vi "Image-DO with Stage - Main_v1.vi"() -> ()   [LabVIEW 2021]
doc: "This program was written by Dr. Michael Everly in support of the research efforts of Dr. Garth Simpson. It provides integrated data acquisition while scanning of a Newport 3 axis rotation stage.. \n\nHardware Required:\nNewport Corp., ESP300 -- 3 axis translation controller with rotation stages.\nTektronix TDS 30xx Oscilloscope\n\n\nWritten by\n Dr. Michael Everly\n Instrumentation Scientist\n Department of Chemistry\n Purdue University\n West Lafayette, IN 47907\n\nCopyright© 2005, All Rights Reserved"
uses:
  Box/Zhang lab general/Software/Amy Imaging_New/Amy Imaging 12-09-2024/Amy Imaging 12-09-2024/Applications/Image-DO with Stage Scan/Support/Type Defs/Image-DO with Stage - Stage Position.ctl
  Box/Zhang lab general/Software/Amy Imaging_New/Amy Imaging 12-09-2024/Amy Imaging 12-09-2024/Applications/Image-DO with Stage Scan/Support/Type Defs/Image-DO with Stage - Imaging Parameters GUI.ctl
  Box/Zhang lab general/Software/Amy Imaging_New/Amy Imaging 12-09-2024/Amy Imaging 12-09-2024/Common/Amy Imager/Type Defs/Imager - Scan Pattern.ctl
  Box/Zhang lab general/Software/Amy Imaging_New/Amy Imaging 12-09-2024/Amy Imaging 12-09-2024/Common/Amy Imager/Type Defs/Imager - Axis Parameters.ctl
  Box/Zhang lab general/Software/Amy Imaging_New/Amy Imaging 12-09-2024/Amy Imaging 12-09-2024/Applications/Image-DO with Stage Scan/Support/Type Defs/Image-DO with Stage - Stage Parameters-Random GUI.ctl
  Box/Zhang lab general/Software/Amy Imaging_New/Amy Imaging 12-09-2024/Amy Imaging 12-09-2024/Applications/Image-DO with Stage Scan/Support/Type Defs/Image-DO with Stage - XY Stage Parameters.ctl
  Box/Zhang lab general/Software/Amy Imaging_New/Amy Imaging 12-09-2024/Amy Imaging 12-09-2024/Applications/Image-DO with Stage Scan/Support/Type Defs/Image-DO with Stage - Z Stage Parameters.ctl
  Box/Zhang lab general/Software/Amy Imaging_New/Amy Imaging 12-09-2024/Amy Imaging 12-09-2024/Applications/Image-DO with Stage Scan/Support/Program Ctrl/Image-DO with Stage - Exec Que.ctl
  Box/Zhang lab general/Software/Amy Imaging_New/Amy Imaging 12-09-2024/Amy Imaging 12-09-2024/Applications/Image-DO with Stage Scan/Support/Program Ctrl/Image-DO with Stage - Exec States.ctl
  Box/Zhang lab general/Software/Amy Imaging_New/Amy Imaging 12-09-2024/Amy Imaging 12-09-2024/Applications/Image-DO with Stage Scan/Support/Program Ctrl/Image-DO with Stage - Sys State.ctl
  <vilib>/Utility/miscctls.llb/LVRectTypeDef.ctl
  Box/Zhang lab general/Software/Amy Imaging_New/Amy Imaging 12-09-2024/Amy Imaging 12-09-2024/Applications/Image-DO with Stage Scan/Support/Type Defs/Image-DO with Stage - File Save Option.ctl
  Box/Zhang lab general/Software/Amy Imaging_New/Amy Imaging 12-09-2024/Amy Imaging 12-09-2024/Applications/Image-DO with Stage Scan/Support/Type Defs/Image-DO with Stage - XYZ Stage Parameters.ctl
  Box/Zhang lab general/Software/Amy Imaging_New/Amy Imaging 12-09-2024/Amy Imaging 12-09-2024/Common/Amy Imager/Type Defs/Imager - AO Scan Settings.ctl
  Box/Zhang lab general/Software/Amy Imaging_New/Amy Imaging 12-09-2024/Amy Imaging 12-09-2024/Common/Amy Imager/Type Defs/Imager - Scan Starting Point.ctl
  <vilib>/Utility/error.llb/DialogType.ctl
  <vilib>/numeric/Random Number (Range) DBL.vi
  <vilib>/Platform/browser.llb/Open URL in Default Browser (string).vi
panel:
  in  "Amy URL":string="Amy Instrument Facility "
  in  "Exit":bool
  in  "Main Tab":enum32{"I/O Config", "Image"}(tab)
  in  "DAQmx Static DO Lines":tag="Dev1/port1/line0:2"
  in  "Y-Mirror DAQmx AO Channel":tag="Dev1/ao1"
  in  "X-Mirror DAQmx AO Channel":tag="Dev1/ao0"
  in  "DAQmx DO Port":tag="Dev1/port0"
  in  "DAQmx AI Channels":T1(array[cluster])=[{"DAQmx AI Channel"="Dev1/ai0", "Channel/Image Name"="Sample"}, {"DAQmx AI Channel"="Dev1/ai1", "Channel/Image Name"="Reference"}]
  in  "Max Value":dbl=1.0 format="%0.2f"
  in  "Min Value":dbl format="%0.2f"
  in  "Prior Stage VISA Resource":refnum<visa-resource-name>="COM1"
  in  "Connect":bool
  in  "Save Masks":bool
  in  "Common Mask":bool caption="Use Common Mask"
  in  "Get Masks":bool
  in  "Scan":bool
  in  "Get Image Mask":bool
  in  "Aquire Image":bool
  in  "Save Image":bool
  in  "Auto Save":bool
  in  "Path":path
  in  "Base Filename":string
  in  "Advance":bool
  in  "Images":dbl[][][](array[numeric])
  in  "Operation":enum32{"Imaging", "Stage Scan"}(tab)
  in  "Imageing Parameters":T2={"Sample Rate"=1000000.0, "Pattern"=enum."Unidirectional Raster", "X Mirror"={"# Pixels"=512, "Center"=0.0, "Span"=0.1, "# Points / Pixel"=10, "Pre-Line pts"=10, "Post-Line pts"=10}, "Y Mirror"={"# Pixels"=512, "Center"=0.0, "Span"=0.1, "# Points / Pixel"=1, "Pre-Line pts"=10, "Post-Line pts"=0}, "Averaged"=TRUE, "Active DO lines"={"Pixel Pattern Bit (0)"=FALSE, "Change Pixel Bit (1)"=FALSE, "New Line Bit (2)"=FALSE, "In Image Bit (3)"=FALSE, "Image Pattern Bits (4-7)"=FALSE}, "Statice DO"=[FALSE, FALSE, FALSE, FALSE, FALSE, FALSE, FALSE, FALSE]} caption="Imaging Parameters" {"Y Mirror"."Post-Line pts" min=0; "Y Mirror"."Pre-Line pts" min=0; "Y Mirror"."# Points / Pixel" min=1; "Y Mirror"."Span" min=0.0 max=0.0 format="%.3f"; "Y Mirror"."Center" format="%.3f"; "Y Mirror"."# Pixels" min=2; "X Mirror"."Post-Line pts" min=0; "X Mirror"."Pre-Line pts" min=0; "X Mirror"."# Points / Pixel" min=1; "X Mirror"."Span" min=0.0 max=0.0 format="%.3f"; "X Mirror"."Center" format="%.3f"; "X Mirror"."# Pixels" min=2}
  out "Estmated Frame Time":dbl caption="Estmated Time: Image / Frame" min=0.0 max=0.0 format="%.1f"
  in  "Cycle Time (sec)":dbl caption="Center" format="%.1f"
  in  "Dwell Time (sec)":dbl caption="Center" format="%.1f"
  in  "User Defined Points":T5={"Step Position"={"X Pos"=0.0, "Y Pos"=0.0, "Z Pos"=0.0}, "Status"="Empty", "First"=FALSE, "Back"=FALSE, "Next"=FALSE, "Last"=FALSE, "Insert Current"=FALSE, "Go To"=FALSE, "Delete"=FALSE, "Clear"=FALSE, "New Position"={"X Pos"=0.0, "Y Pos"=0.0, "Z Pos"=0.0}, "Insert"=FALSE} {"Step Position"."X Pos" format="%.1f"; "Step Position"."Y Pos" format="%.1f"; "Step Position"."Z Pos" format="%.1f"; "New Position"."X Pos" format="%.1f"; "New Position"."Y Pos" format="%.1f"; "New Position"."Z Pos" format="%.1f"}
  in  "Grid Parameters":T7={"X Axis"={"Start Pt"=0.0, "Step Size"=100.0, "# Steps"=12}, "Y Axis"={"Start Pt"=20.0, "Step Size"=2.0, "# Steps"=2}, "Pattern"=enum."Bidirectional Raster", "Major Axis"=FALSE} caption="X Axis" {"X Axis"."Step Size" format="%.1f"; "X Axis"."Start Pt" format="%.1f"; "X Axis"."# Steps" min=1 step=1; "Y Axis"."Step Size" format="%.1f"; "Y Axis"."Start Pt" format="%.1f"; "Y Axis"."# Steps" min=1 step=1}
  in  "XY Scan Mode":bool caption="Z Axis"
  in  "Z Scan Parameters":T8={"Z Axis"={"Start Pt"=100.0, "Step Size"=20.0, "# Steps"=0}, "Pattern"=enum."Unidirectional Raster", "Active"=FALSE} caption="X Axis" {"Z Axis"."Step Size" format="%.1f"; "Z Axis"."Start Pt" format="%.1f"; "Z Axis"."# Steps" min=1 step=1}
  in  "Step Mode":bool
  in  "Row #":dbl(c297)
  out "Status":string
  out "Current Position":T6 caption="Stage Position" {"X Pos" format="%.1f"; "Y Pos" format="%.1f"; "Z Pos" format="%.1f"}
  in  "Reset I/O":bool
  in  "Get Position":bool
  in  "Go Home Prior":bool
  in  "Set Home Prior":bool
  # "Static Digital Control Lines"
  # "Mirror Control"
  # "Digital / Mask Control"
  # "Image / Data Acquisition"
  # "Stage Control"
  # "Stage Scanning"
  # "Image Scanning"
  # "1         line #         8"
  # "Scanning Parameters"
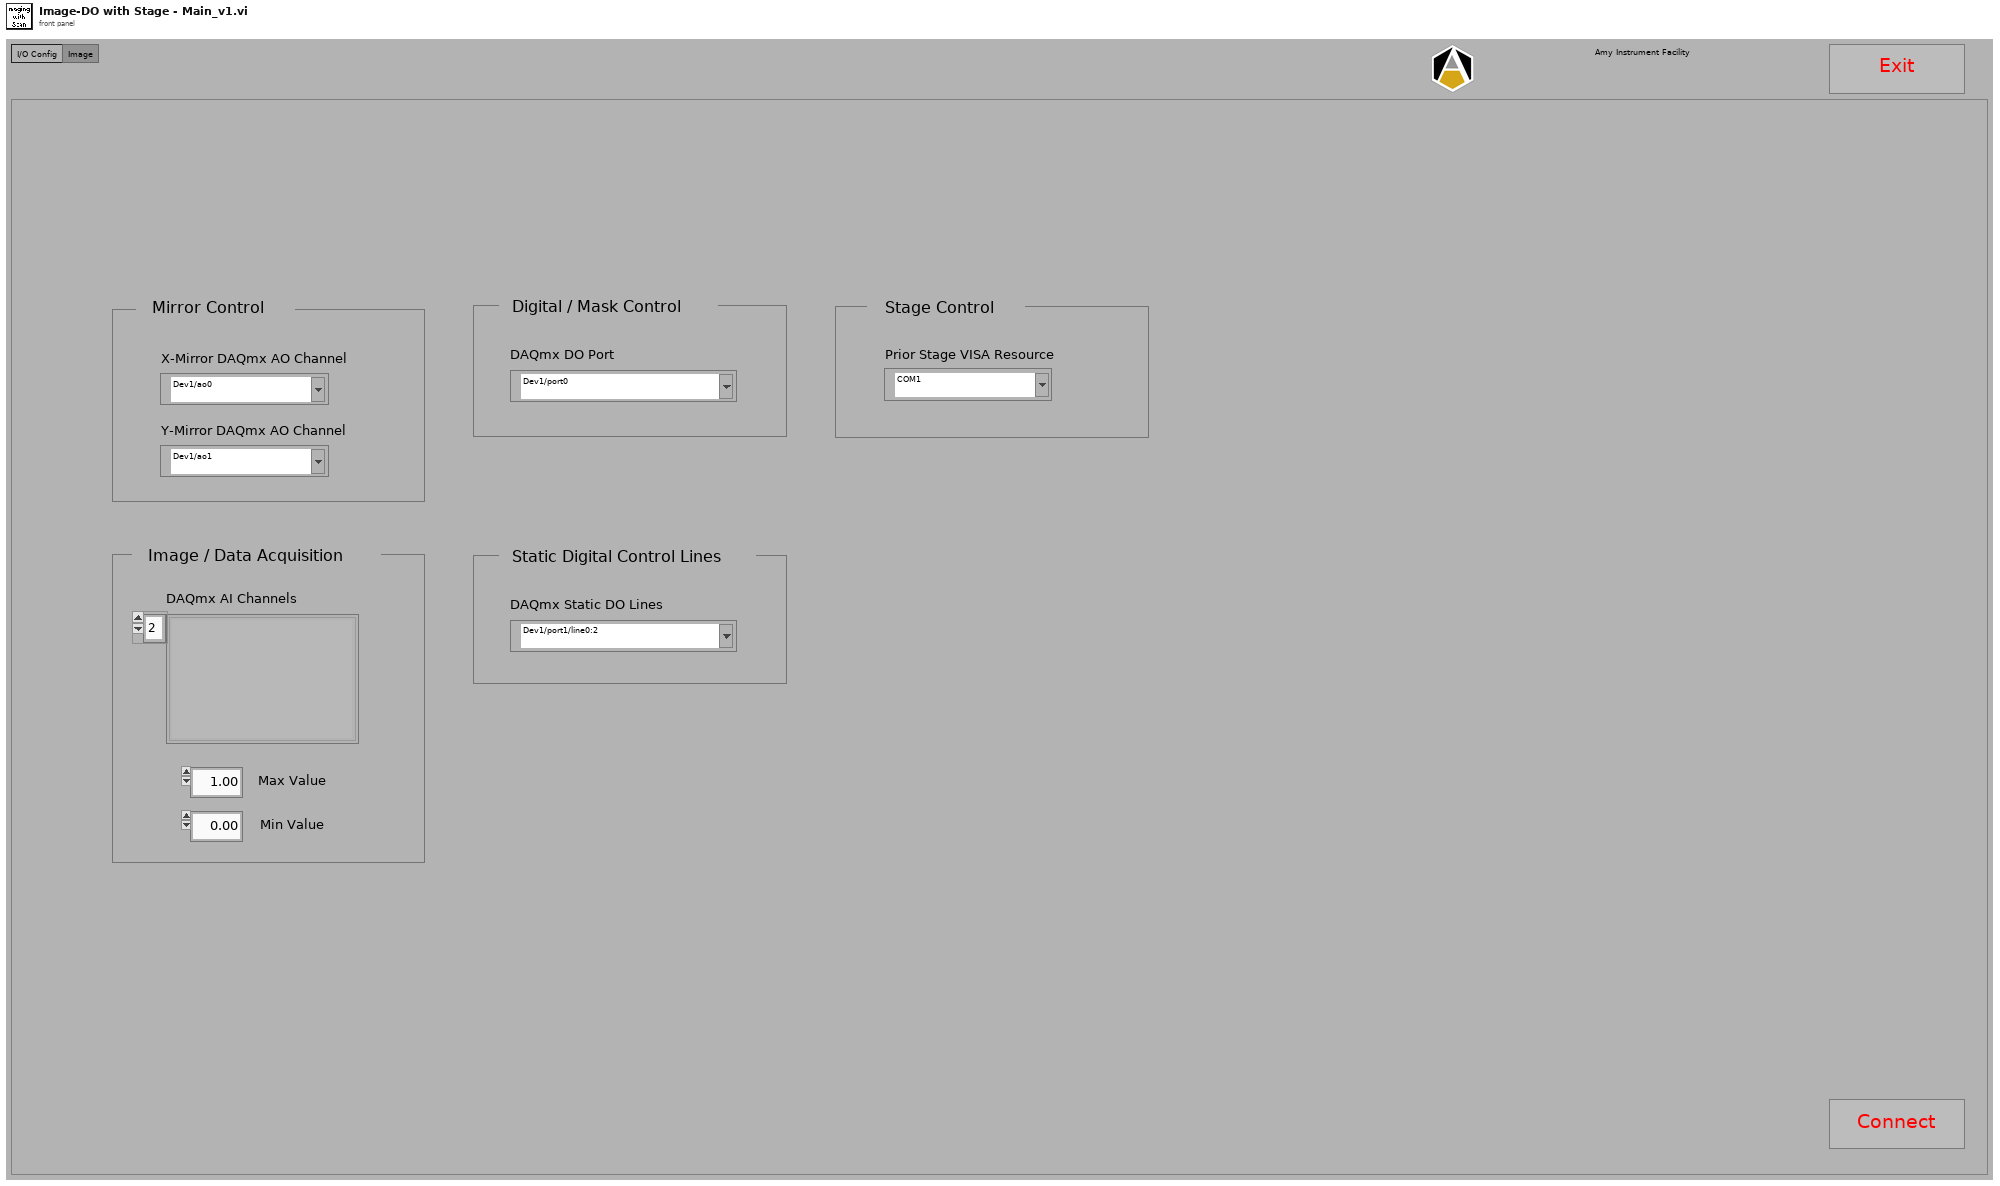
[diagram p1: front panel]
types:
  T1 = cluster{"DAQmx AI Channel":tag, "Channel/Image Name":string}[]
  T2 = typedef "Image-DO with Stage - Imaging Parameters GUI.ctl" = cluster{"Sample Rate":dbl, "Pattern":T3, "X Mirror":T4, "Y Mirror":T4, "Averaged":bool, "Active DO lines":cluster{"Pixel Pattern Bit (0)":bool, "Change Pixel Bit (1)":bool, "New Line Bit (2)":bool, "In Image Bit (3)":bool, "Image Pattern Bits (4-7)":bool}, "Statice DO":bool[]}
  T3 = typedef "Imager - Scan Pattern.ctl" = enum16{"Unidirectional Raster", "Bidirectional Raster"}
  T4 = typedef "Imager - Axis Parameters.ctl" = cluster{"# Pixels":i32, "Center":dbl, "Span":dbl, "# Points / Pixel":i32, "Pre-Line pts":i32, "Post-Line pts":i32}
  T5 = typedef "Image-DO with Stage - Stage Parameters-Random GUI.ctl" = cluster{"Step Position":T6, "Status":string, "First":bool, "Back":bool, "Next":bool, "Last":bool, "Insert Current":bool, "Go To":bool, "Delete":bool, "Clear":bool, "New Position":T6, "Insert":bool}
  T6 = typedef "Image-DO with Stage - Stage Position.ctl" = cluster{"X Pos":dbl, "Y Pos":dbl, "Z Pos":dbl}
  T7 = typedef "Image-DO with Stage - XY Stage Parameters.ctl" = cluster{"X Axis":cluster{"Start Pt":dbl, "Step Size":dbl, "# Steps":i32}, "Y Axis":cluster{"Start Pt":dbl, "Step Size":dbl, "# Steps":i32}, "Pattern":enum16{"Unidirectional Raster", "Bidirectional Raster"}, "Major Axis":bool}
  T8 = typedef "Image-DO with Stage - Z Stage Parameters.ctl" = cluster{"Z Axis":cluster{"Start Pt":dbl, "Step Size":dbl, "# Steps":i32}, "Pattern":enum16{"Unidirectional Raster", "Bidirectional Raster"}, "Active":bool}
  T9 = typedef "Image-DO with Stage - Exec Que.ctl" = cluster{"Exec States":T10, "U32":u32, "I32":i32, "DBL_1 (X)":dbl, "DBL_2 (Y)":dbl, "DBL_3 (Z)":dbl, "Bool_1":bool, "Bool_2":bool, "Variant":variant}
  T10 = typedef "Image-DO with Stage - Exec States.ctl" = enum16{"SW Init", "HW Init Ctrl", "HW Init - DAQmx", "HW Init - Prior", "HW Init - Reserve 1", "HW Init - Reserve 2", "HW Init - SW", "Pre-Image Crtl", "Pre-Image HW - DAQmx", "Pre-Image HW - Prior", "Pre-Image HW - Reserve 1", "Pre-Image HW - Reserve 2", "Pre-Image SW", "Image Ctrl", "Post-Image Crtl", "Post-Image HW - DAQmx", "Post-Image HW - Prior", "Post-Image HW - Reserve 1", "Post-Image HW - Reserve 2", "Post-Image SW", "Pre-Mask Ctrl", "Pre-Mask HW - DAQmx", "Pre-Mask HW - Prior", "Pre-Mask HW - Reserved 1", "Pre-Mask HW - Reserved 2", "Pre-Mask SW", "Mask Crtl", "Post-Mask Crtl", "Post-Mask HW - DAQmx", "Post-Mask HW - Prior", "Post-Mask HW - Reserved 1", "Post-Mask HW - Reserved 2", "Post-Mask SW", "Pre-Scan Ctrl", "Pre-Scan HW - DAQmx", "Pre-Scan HW - Prior", "Pre-Scan HW - Reserve 1", "Pre-Scan HW - Reserve 2", "Pre-Scan SW", "Scan Ctrl", "Post-Scan Crtl", "Post-Scan HW - DAQmx", "Post-Scan HW - Prior", "Post-Scan HW - Reserve 1", "Post-Scan HW - Reserve 2", "Post-Scan SW", "Wait (ms)", "Confgure Imaging - DAQmx", "Start Imaging - DAQmx", "Read Images - DAQmx", "Wait on Image Complete - DAQmx", "Stop Imaging - DAQmx", "Set Position - Prior", "Get Position - Prior", "Wait on Move Complete - Prior", "Process Data", "Display Image", "Display Scan", "Save Files", "Wait on User", "Update Mask", "Reserved 3", "Reserved 4", "Reserved 5", "HW Close Crtl", "HW Close - DAQmx", "HW Close - Prior", "HW Close - Reserve 1", "HW Close - Reserve 2", "HW Close - SW", "Shutdown", "Error", "Exit"}
  T11 = enum16{"Get All", "Set Path", "Set Filename", "Set Descriptor", "Set Image Settings", "Set Stage Settings", "Set # XY Points"}
  T12 = typedef "Image-DO with Stage - Sys State.ctl" = enum16{"HW Un_init", "HW Initializing", "HW Initialized", "Configuring", "Configured", "Imaging", "Masking", "Scanning"}
  T13 = cluster{"Exec States":u16, "U32":u32, "I32":i32, "DBL_1 (X)":dbl, "DBL_2 (Y)":dbl, "DBL_3 (Z)":dbl, "Bool_1":bool, "Bool_2":bool, "Variant":variant}[]
  T14 = enum16{"Read", "Go to First", "Step Forward", "Step Back", "Go to Last", "Insert", "Delete", "Delete All", "Insert Pts in"}
  T15 = typedef "Image-DO with Stage - File Save Option.ctl" = enum16{"Save Image Parameters", "Save Scan Parameters", "Save Mask", "Save Image", "Open Data Files", "Append Data Files", "Close Data Files"}
  T16 = typedef "Image-DO with Stage - Imaging Settings.ctl" = cluster{"DAQmx AI Channels":tag[], "Channel Names":string[], "Sample Rate":dbl, "Pattern":T3, "Starting Pt":T17, "X Mirror":T4, "Y Mirror":T4, "Averaged Data":bool}
  T17 = typedef "Imager - Scan Starting Point.ctl" = enum16{"X-Min, Y-Min", "X-Min, Y-Max", "X-Max, Y-Min", "X-Max, Y-Max"}
  T18 = cluster{"Step Position":cluster{"X Pos":bool, "Y Pos":bool, "Z Pos":bool}, "Status":bool, "First":bool, "Back":bool, "Next":bool, "Last":bool, "Insert Current":bool, "Go To":bool, "Delete":bool, "Clear":bool, "New Position":cluster{"X Pos":bool, "Y Pos":bool, "Z Pos":bool}, "Insert":bool}
  T19 = enum16{"Get All Mask", "Set Imaging Mask", "Init Scan Masks", "Get Scan Mask (n)", "Set Scan Mask (n)", "Set Scan Masks"}
  T20 = typedef "LVRectTypeDef.ctl" = cluster{"Left":i16, "Top":i16, "Right":i16, "Bottom":i16}
  T21 = enum16{"Create Task", "Write Lnes", "Clear Task"}
  T22 = enum16{"Get Current", "Go Home/First", "Step Forward", "Step Back", "Go To #", "Load Points"}
  T23 = typedef "Image-DO with Stage - XYZ Stage Parameters.ctl" = cluster{"Grid":T7, "Z Scan":T8, "XY Scan Mode":bool, "Dwell Time":dbl, "Cycle Time":dbl}
  T24 = typedef "Imager - AO Scan Settings.ctl" = cluster{"Sample Rate":dbl, "Pattern":T3, "Starting Pt":T17, "X Mirror":T4, "Y Mirror":T4}
  T25 = cluster{"DO Port Map":cluster{"Pixel Pattern Bit (0)":u8, "Change Pixel Bit (1)":u8, "New Line Bit (2)":u8, "In Image Bit (3)":u8, "Image Pattern Bits (4-7)":u8}, "Active DO lines":cluster{"Pixel Pattern Bit (0)":bool, "Change Pixel Bit (1)":bool, "New Line Bit (2)":bool, "In Image Bit (3)":bool, "Image Pattern Bits (4-7)":bool}, "Pixel Mask":u8[][], "Image Mask":u8[][]}
  T26 = cluster{"X Axis":dbl, "Y Axis":dbl, "Z Axis":dbl}
  T27 = enum16{"Do not append", "Current File", "Alternate File"}
  T28 = typedef "Image-DO with Stage - Scan Step Info.ctl" = cluster{"# X Steps":i32, "# Y Steps":i32, "# Z Steps":i32, "# XY Steps":i32, "# Total Steps":i32, "X Step #":i32, "Y Step #":i32, "Z Step #":i32, "XY Step #":i32, "Total Step #":i32}
  T29 = cluster{"# XY Steps":i32, "# Pixels":i32, "# Pixels":i32}
  T30 = cluster{"Pixel Pattern Bit (0)":bool, "Change Pixel Bit (1)":bool, "New Line Bit (2)":bool, "In Image Bit (3)":bool, "Image Pattern Bits (4-7)":bool}
  T31 = typedef "DialogType.ctl" = u16
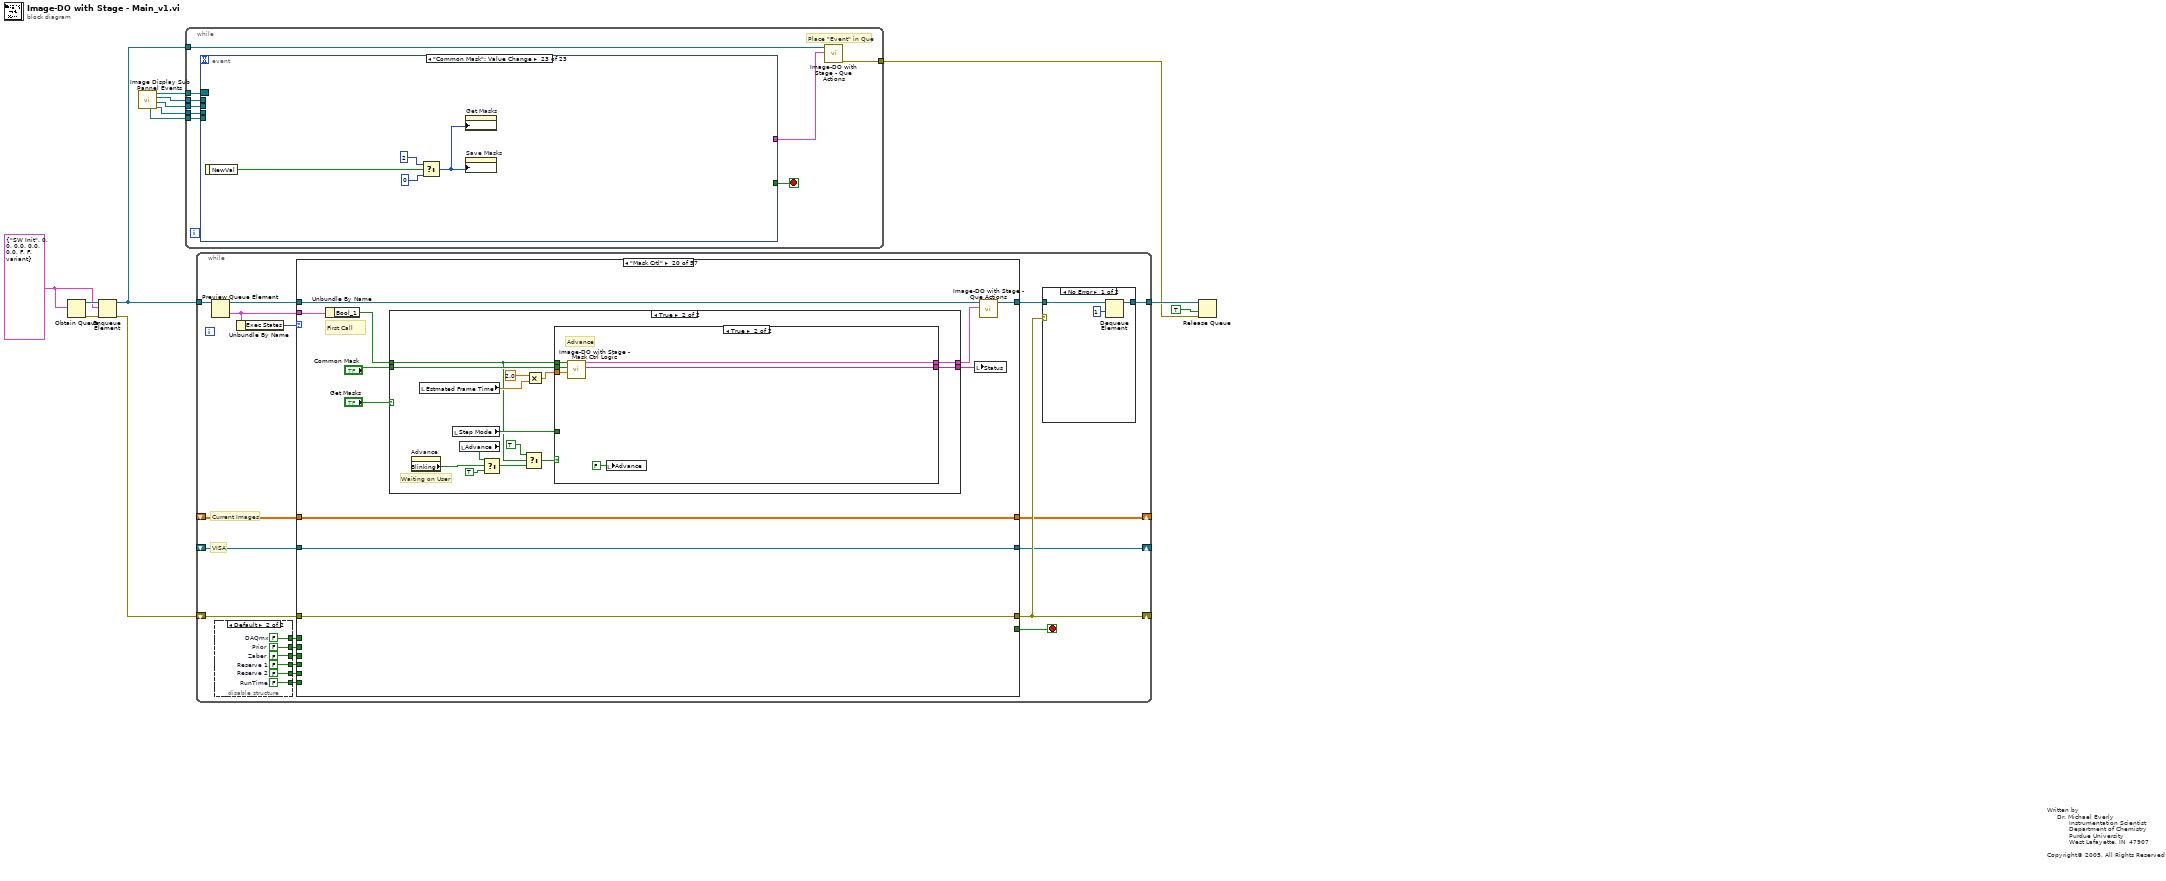
[diagram p0: block diagram]
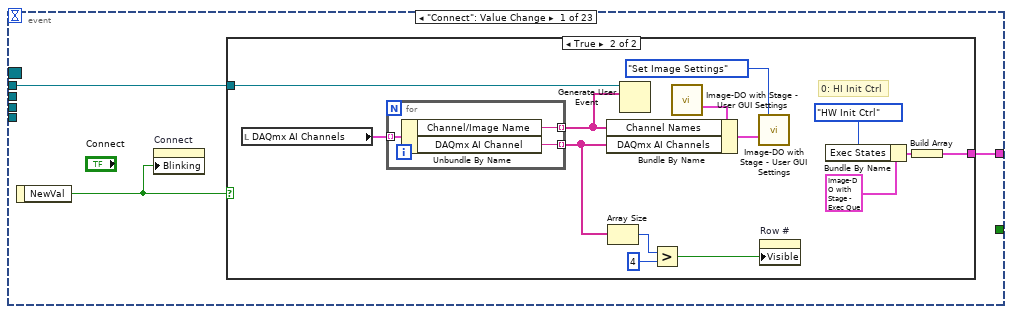
[diagram p2: hidden frame]
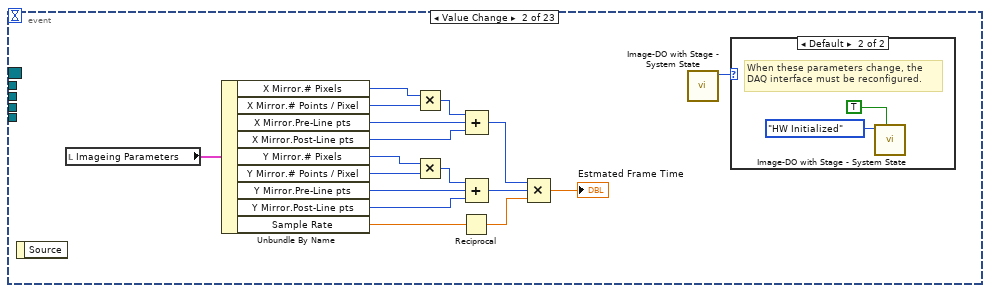
[diagram p4: hidden frame]
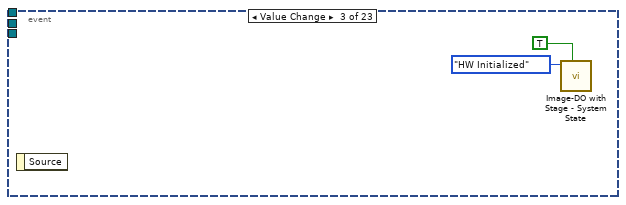
[diagram p6: hidden frame]
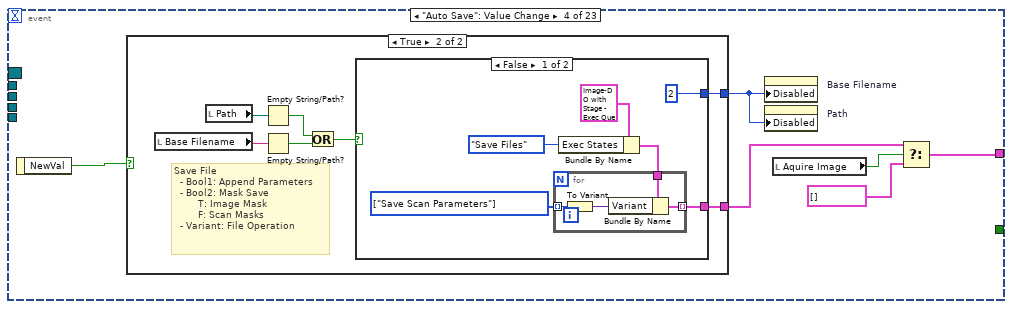
[diagram p7: hidden frame]
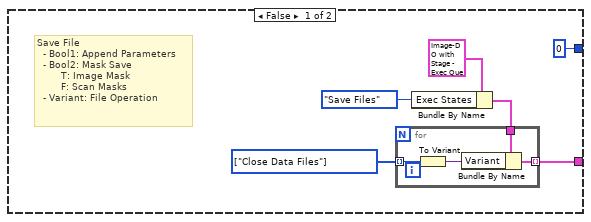
[diagram p8: hidden frame]
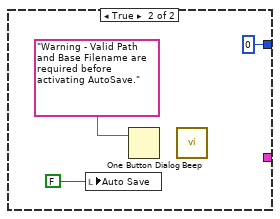
[diagram p9: hidden frame]
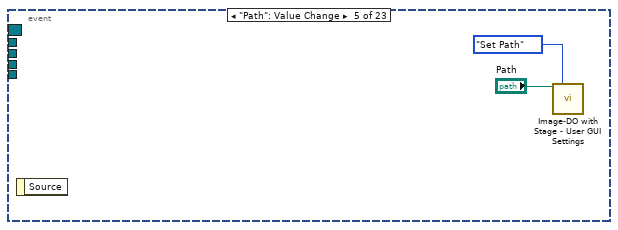
[diagram p10: hidden frame]
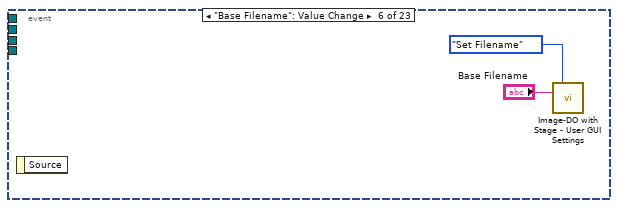
[diagram p11: hidden frame]
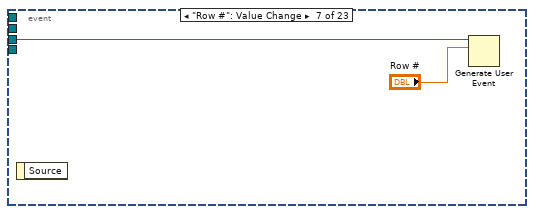
[diagram p12: hidden frame]
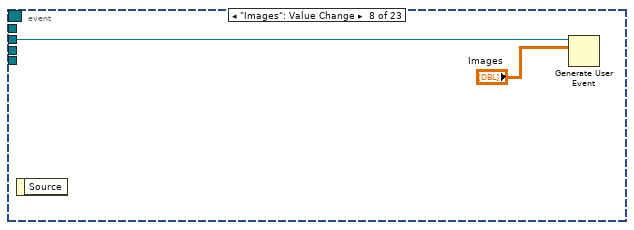
[diagram p13: hidden frame]
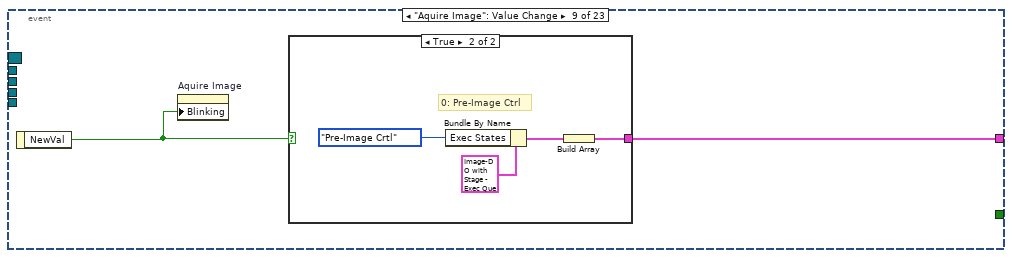
[diagram p14: hidden frame]
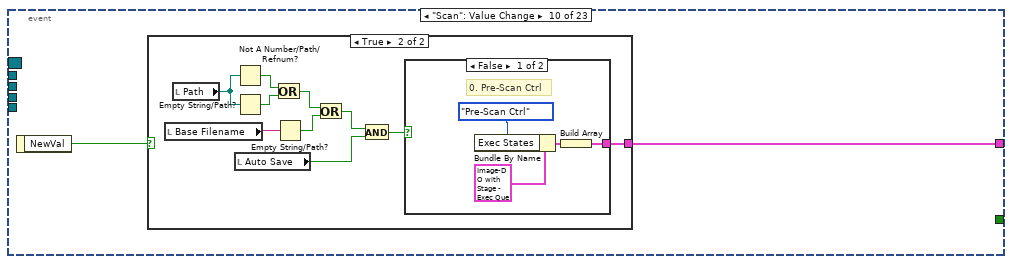
[diagram p16: hidden frame]
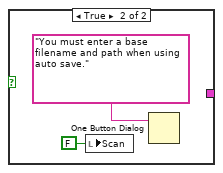
[diagram p18: hidden frame]
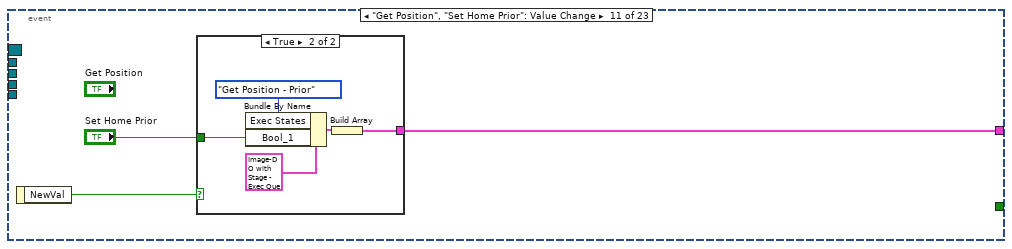
[diagram p19: hidden frame]
diagram:
  w9 = T9 {"Exec States"=enum."SW Init", "U32"=0, "I32"=0, "DBL_1 (X)"=0.0, "DBL_2 (Y)"=0.0, "DBL_3 (Z)"=0.0, "Bool_1"=FALSE, "Bool_2"=FALSE, "Variant"=variant(string "")}
  # "Written by\n     Dr. Michael Everly\n           Instrumentation Scientist\n           Department of Chemistry\n           Purdue University\n           West Lafayette, IN  47907\n\nCopyright© 2005, All Rights Reserved"
  n1 = Obtain Queue(element data type=w9) -> (queue out=w12:refnum<queue>, error out=w13:errorcluster)  [unwired: 4 in, 1 out]
  n2 = Enqueue Element(queue=w12, element=w9, error in (no error)=w13) -> (queue out=w10:refnum<queue>, error out=w11:errorcluster)  [unwired: 1 in, 1 out]
  n3 = call "Image Display Sub Pannel Events.vi"() -> ("Row # user event"=w2:refnum<user-event>, "Data user event"=w3:refnum<user-event>, "Captions user event"=w4:refnum<user-event>, "Event Registration Refnum"=w5:refnum<event-registration>, "Exit event out"=w1:refnum<user-event>)  [unwired: 7 in]
  n4 = while {
    tunnel: w10 -> [w21]
    tunnel: [w20] -> w6
    tunnel: w5 -> [w18]
    tunnel: w4 -> [w17]
    tunnel: w3 -> [w16]
    tunnel: w2 -> [w15]
    tunnel: w1 -> [w14]
    stop <- w19 stop-if-true
    # "Place \"Event\" in Que"
    n5 = event shown="[22] \"Common Mask\": Value Change" {
      selector: w18 -> [_ _ _ _ _ _ _ _ _ _ _ _ _ _ _ _ _ _ _ _ _ _ _]
      dyn-events: _ -> [_ _ _ _ _ _ _ _ _ _ _ _ _ _ _ _ _ _ _ _ _ _ _]
      timeout: _ -> [_ _ _ _ _ _ _ _ _ _ _ _ _ _ _ _ _ _ _ _ _ _ _]
      tunnel: [w25 _ _ w65 _ _ _ _ w108 w115 w134 w141 w151 w158 w167 _ _ _ w188 w248 w254 w261 _] -> w22
      tunnel: [_ _ _ _ _ _ _ _ _ _ _ _ _ _ w166 _ _ _ _ _ _ _ _] -> w19
      tunnel: w17 -> [w23 _ _ _ _ _ _ _ _ _ _ _ _ _ _ _ _ _ _ _ _ _ _]
      tunnel: w16 -> [_ _ _ _ _ _ _ w107 _ _ _ _ _ _ _ _ _ _ _ _ _ _ _]
      tunnel: w15 -> [_ _ _ _ _ _ w105 _ _ _ _ _ _ _ _ _ _ _ _ _ _ _ _]
      tunnel: w14 -> [_ _ _ _ _ _ _ _ _ _ _ _ _ _ w168 _ _ _ _ _ _ _ _]
      event "Connect": Value Change {
        n6 = event-data() -> ("NewVal"=w24:bool)  [unwired: 1 in]
        n7 = property on="Connect" class="Bool (strict)"("Blinking"=w24) -> ()  [unwired: 2 in, 2 out]
        n8 = case shown="True" w24 {
          tunnel: [_ w36] -> w25
          tunnel: w23 -> [_ w35]
          frame False {
          }
          frame True {
            # "0: HI Init Ctrl"
            n9 = local read "DAQmx AI Channels"() -> (w34:T1)
            n10 = for {
              tunnel: w34 -> [w42] mode=indexing
              tunnel: [w41] -> w33 mode=indexing
              tunnel: [w40] -> w30 mode=indexing
              n11 = Unbundle By Name(w42) -> ("Channel/Image Name"=w41:string, "DAQmx AI Channel"=w40:tag)
            }
            n12 = Array Size(array=w30) -> (size(s)=w32:i32)
            n13 = Generate User Event(user event=w35, event data cluster=w33) -> ()  [unwired: 2 in, 2 out]
            n14 = Greater?(x=w32, y=4) -> (0:w29:bool)
            n15 = call "Image-DO with Stage - User GUI Settings.vi"() -> ("Imaging Settings Out"=w27:T16)  [unwired: 10 in, 5 out]
            n16 = Bundle By Name(cluster=w27, "Channel Names"=w33, "DAQmx AI Channels"=w30) -> (w26:T16)
            n17 = call "Image-DO with Stage - User GUI Settings.vi"("Action (0: Read All)"=T11."Set Image Settings", "Imaging Settings In"=w26) -> ()  [unwired: 8 in, 6 out]
            n18 = property on="Row #" class="Scroll (strict)"("Visible"=w29) -> ()  [unwired: 2 in, 2 out]
            n19 = Bundle By Name(cluster=T9 {"Exec States"=enum."SW Init", "U32"=0, "I32"=0, "DBL_1 (X)"=0.0, "DBL_2 (Y)"=0.0, "DBL_3 (Z)"=0.0, "Bool_1"=FALSE, "Bool_2"=FALSE, "Variant"=variant(string "")} ("Que"), "Exec States"=Image-DO_with_Stage_-_Exec_States."HW Init Ctrl") -> (w39:T9)
            n20 = Build Array(w39) -> (w36:T9[])
          }
        }
      }
      event Value Change {
        n21 = event-data() -> ()  [unwired: 1 in, 1 out]
        n22 = local read "Imageing Parameters"() -> (w49:T2)
        n23 = Unbundle By Name(w49) -> ("X Mirror.# Pixels"=w51:i32, "X Mirror.# Points / Pixel"=w59:i32, "X Mirror.Pre-Line pts"=w57:i32, "X Mirror.Post-Line pts"=w56:i32, "Y Mirror.# Pixels"=w48:i32, "Y Mirror.# Points / Pixel"=w47:i32, "Y Mirror.Pre-Line pts"=w46:i32, "Y Mirror.Post-Line pts"=w45:i32, "Sample Rate"=w44:dbl)
        n24 = Multiply(x=w51, y=w59) -> (x*y=w58:i32)
        n25 = Multiply(x=w48, y=w47) -> (x*y=w55:i32)
        n26 = Reciprocal(x=w44) -> (1/x=w52:dbl)
        n27 = Compound Arithmetic op=ADD(w58, w57, w56) -> (w54:i32)
        n28 = Compound Arithmetic op=ADD(w55, w46, w45) -> (w53:i32)
        n29 = Compound Arithmetic op=MULTIPLY(w54, w53, w52) -> (→"Estmated Frame Time":dbl)
        n30 = call "Image-DO with Stage - System State.vi"() -> ("Sys State Out"=w43:T12)  [unwired: 9 in, 2 out]
        n31 = case shown="Default" w43 {
          frame "HW Un_init" {
          }
          frame Default {
            # "When these parameters change, the \nDAQ interface must be reconfigured."
            n32 = call "Image-DO with Stage - System State.vi"("Set State (F:Get)"=TRUE ("Action (F:Get)"), "Sys State In"=Image-DO_with_Stage_-_Sys_State."HW Initialized") -> ()  [unwired: 7 in, 3 out]
          }
        }
      }
      event Value Change {
        n33 = event-data() -> ()  [unwired: 1 in, 1 out]
        n34 = call "Image-DO with Stage - System State.vi"("Set State (F:Get)"=TRUE ("Action (F:Get)"), "Sys State In"=Image-DO_with_Stage_-_Sys_State."HW Initialized") -> ()  [unwired: 7 in, 3 out]
      }
      event "Auto Save": Value Change {
        n35 = event-data() -> ("NewVal"=w69:bool)  [unwired: 1 in]
        n36 = case shown="True" w69 {
          tunnel: [w71 w83] -> w67
          tunnel: [u8 0 ("Disabled") w80] -> w64
          frame False {
            w74 = T15[] [enum."Close Data Files"] items=["Save Image Parameters", "Save Scan Parameters", "Save Mask", "Save Image", "Open Data Files", "Append Data Files", "Close Data Files"]
            # "Save File\n  - Bool1: Append Parameters\n  - Bool2: Mask Save\n        T: Image Mask\n        F: Scan Masks\n  - Variant: File Operation"
            n37 = Bundle By Name(cluster=T9 {"Exec States"=enum."SW Init", "U32"=0, "I32"=0, "DBL_1 (X)"=0.0, "DBL_2 (Y)"=0.0, "DBL_3 (Z)"=0.0, "Bool_1"=FALSE, "Bool_2"=FALSE, "Variant"=variant(string "")} ("Que"), "Exec States"=Image-DO_with_Stage_-_Exec_States."Save Files") -> (w75:T9)
            n38 = for {
              tunnel: w75 -> [w79]
              tunnel: w74 -> [w77] mode=indexing
              tunnel: [w76] -> w71 mode=indexing
              n39 = To Variant(anything=w77) -> (Variant=w78:variant)
              n40 = Bundle By Name(cluster=w79, "Variant"=w78) -> (w76:T9)
            }
          }
          frame True {
            # "Save File\n  - Bool1: Append Parameters\n  - Bool2: Mask Save\n        T: Image Mask\n        F: Scan Masks\n  - Variant: File Operation"
            n41 = local read "Base Filename"() -> (w81:string)
            n42 = local read "Path"() -> (w82:path)
            n43 = Empty String/Path?(string/path=w82) -> (empty?=w85:bool)
            n44 = Empty String/Path?(string/path=w81) -> (empty?=w84:bool)
            n45 = Or(x=w85, y=w84) -> (x .or. y?=w86:bool)
            n46 = case shown="False" w86 {
              tunnel: [w88 _] -> w83
              tunnel: [u8 2 ("Disabled") u8 0 ("Disabled")] -> w80
              frame False {
                w91 = T15[] [enum."Save Scan Parameters"] items=["Save Image Parameters", "Save Scan Parameters", "Save Mask", "Save Image", "Open Data Files", "Append Data Files", "Close Data Files"]
                n47 = Bundle By Name(cluster=T9 {"Exec States"=enum."SW Init", "U32"=0, "I32"=0, "DBL_1 (X)"=0.0, "DBL_2 (Y)"=0.0, "DBL_3 (Z)"=0.0, "Bool_1"=FALSE, "Bool_2"=FALSE, "Variant"=variant(string "")} ("Que"), "Exec States"=Image-DO_with_Stage_-_Exec_States."Save Files") -> (w92:T9)
                n48 = for {
                  tunnel: w92 -> [w96]
                  tunnel: w91 -> [w94] mode=indexing
                  tunnel: [w93] -> w88 mode=indexing
                  n49 = To Variant(anything=w94) -> (Variant=w95:variant)
                  n50 = Bundle By Name(cluster=w96, "Variant"=w95) -> (w93:T9)
                }
              }
              frame True {
                n51 = local write "Auto Save"(FALSE ("Auto Save")) -> ()
                n52 = One Button Dialog(message="Warning - Valid Path and Base Filename are required before activating AutoSave.") -> ()  [unwired: 1 in, 1 out]
                n53 = call <vilib>:"Beep.vi"() -> ()  [unwired: 12 in]
              }
            }
          }
        }
        n54 = property on="Base Filename" class="Str"("Disabled"=w64) -> ()  [unwired: 2 in, 2 out]
        n55 = property on="Path" class="Path"("Disabled"=w64) -> ()  [unwired: 2 in, 2 out]
        n56 = local read "Aquire Image"() -> (w68:bool)
        n57 = Select(t=w67, s=w68, f=T13 []) -> (s? t:f=w65:T13)
      }
      event "Path": Value Change {
        n58 = event-data() -> ()  [unwired: 1 in, 1 out]
        n59 = call "Image-DO with Stage - User GUI Settings.vi"("Path In"="Path", "Action (0: Read All)"=T11."Set Path") -> ()  [unwired: 8 in, 6 out]
      }
      event "Base Filename": Value Change {
        n60 = event-data() -> ()  [unwired: 1 in, 1 out]
        n61 = call "Image-DO with Stage - User GUI Settings.vi"("Action (0: Read All)"=T11."Set Filename", "Base Filename In"="Base Filename") -> ()  [unwired: 8 in, 6 out]
      }
      event "Row #": Value Change {
        n62 = event-data() -> ()  [unwired: 1 in, 1 out]
        n63 = Generate User Event(user event=w105, event data cluster="Row #") -> ()  [unwired: 2 in, 2 out]
      }
      event "Images": Value Change {
        n64 = event-data() -> ()  [unwired: 1 in, 1 out]
        n65 = Generate User Event(user event=w107, event data cluster="Images") -> ()  [unwired: 2 in, 2 out]
      }
      event "Aquire Image": Value Change {
        n66 = event-data() -> ("NewVal"=w109:bool)  [unwired: 1 in]
        n67 = property on="Aquire Image" class="Bool (strict)"("Blinking"=w109) -> ()  [unwired: 2 in, 2 out]
        n68 = case shown="True" w109 {
          tunnel: [_ w111] -> w108
          frame False {
          }
          frame True {
            # "0: Pre-Image Ctrl"
            n69 = Bundle By Name(cluster=T9 {"Exec States"=enum."SW Init", "U32"=0, "I32"=0, "DBL_1 (X)"=0.0, "DBL_2 (Y)"=0.0, "DBL_3 (Z)"=0.0, "Bool_1"=FALSE, "Bool_2"=FALSE, "Variant"=variant(string "")} ("Que"), "Exec States"=Image-DO_with_Stage_-_Exec_States."Pre-Image Crtl") -> (w113:T9)
            n70 = Build Array(w113) -> (w111:T9[])
          }
        }
      }
      event "Scan": Value Change {
        n71 = event-data() -> ("NewVal"=w114:bool)  [unwired: 1 in]
        n72 = case shown="True" w114 {
          tunnel: [_ w125] -> w115
          frame False {
          }
          frame True {
            n73 = local read "Base Filename"() -> (w121:string)
            n74 = local read "Path"() -> (w122:path)
            n75 = Not A Number/Path/Refnum?(number/path/refnum=w122) -> (NaN/Path/Refnum?=w124:bool)
            n76 = Empty String/Path?(string/path=w122) -> (empty?=w123:bool)
            n77 = local read "Auto Save"() -> (w117:bool)
            n78 = Or(x=w124, y=w123) -> (x .or. y?=w120:bool)
            n79 = Empty String/Path?(string/path=w121) -> (empty?=w119:bool)
            n80 = Or(x=w120, y=w119) -> (x .or. y?=w118:bool)
            n81 = And(x=w118, y=w117) -> (x .and. y?=w116:bool)
            n82 = case shown="False" w116 {
              tunnel: [w126 _] -> w125
              frame False {
                # "0. Pre-Scan Ctrl"
                n83 = Bundle By Name(cluster=T9 {"Exec States"=enum."SW Init", "U32"=0, "I32"=0, "DBL_1 (X)"=0.0, "DBL_2 (Y)"=0.0, "DBL_3 (Z)"=0.0, "Bool_1"=FALSE, "Bool_2"=FALSE, "Variant"=variant(string "")} ("Que"), "Exec States"=Image-DO_with_Stage_-_Exec_States."Pre-Scan Ctrl") -> (w129:T9)
                n84 = Build Array(w129) -> (w126:T9[])
              }
              frame True {
                n85 = local write "Scan"(FALSE ("Scan")) -> ()
                n86 = One Button Dialog(message="You must enter a base filename and path when using auto save.") -> ()  [unwired: 1 in, 1 out]
              }
            }
          }
        }
      }
      event "Get Position", "Set Home Prior": Value Change {
        n87 = event-data() -> ("NewVal"=w133:bool)  [unwired: 1 in]
        n88 = case shown="True" w133 {
          tunnel: [_ w136] -> w134
          tunnel: "Set Home Prior" -> [_ w135]
          frame False {
          }
          frame True {
            n89 = Bundle By Name(cluster=T9 {"Exec States"=enum."SW Init", "U32"=0, "I32"=0, "DBL_1 (X)"=0.0, "DBL_2 (Y)"=0.0, "DBL_3 (Z)"=0.0, "Bool_1"=FALSE, "Bool_2"=FALSE, "Variant"=variant(string "")} ("Que"), "Exec States"=Image-DO_with_Stage_-_Exec_States."Get Position - Prior", "Bool_1"=w135) -> (w139:T9)
            n90 = Build Array(w139) -> (w136:T9[])
          }
        }
      }
      event "Go Home Prior": Value Change {
        n91 = event-data() -> ("NewVal"=w140:bool)  [unwired: 1 in]
        n92 = case shown="True" w140 {
          tunnel: [_ w147] -> w141
          frame False {
          }
          frame True {
            n93 = local read "Z Scan Parameters"() -> (w143:T8)
            n94 = local read "Grid Parameters"() -> (w144:T7)
            n95 = Unbundle By Name(w144) -> ("X Axis.Start Pt"=w146:dbl, "Y Axis.Start Pt"=w145:dbl)
            n96 = Unbundle By Name(w143) -> ("Z Axis.Start Pt"=w142:dbl)
            n97 = Bundle By Name(cluster=T9 {"Exec States"=enum."SW Init", "U32"=0, "I32"=0, "DBL_1 (X)"=0.0, "DBL_2 (Y)"=0.0, "DBL_3 (Z)"=0.0, "Bool_1"=FALSE, "Bool_2"=FALSE, "Variant"=variant(string "")} ("Que"), "Exec States"=Image-DO_with_Stage_-_Exec_States."Set Position - Prior", "DBL_1 (X)"=w146, "DBL_2 (Y)"=w145, "DBL_3 (Z)"=w142) -> (w150:T9)
            n98 = Build Array(w150) -> (w147:T9[])
          }
        }
      }
      event "Save Image": Value Change {
        n99 = event-data() -> ("NewVal"=w152:bool)  [unwired: 1 in]
        n100 = case shown="True" w152 {
          tunnel: [_ w154] -> w151
          frame False {
          }
          frame True {
            n101 = call "Image-DO with Stage - Select Files.vi"() -> ("error out"=w153:errorcluster, "Actions"=w154:T9[])  [unwired: 10 in]
            n102 = flat-sequence {
              tunnel: w153 -> [_]
              frame #0 {
                n103 = call "Image-DO with Stage - User GUI Settings.vi"() -> ("Path Out"=w156:path, "Base Filename Out"=w155:string)  [unwired: 10 in, 4 out]
                n104 = local write "Path"(w156) -> ()
                n105 = local write "Base Filename"(w155) -> ()
              }
            }
          }
        }
      }
      event "Reset I/O": Value Change {
        n106 = event-data() -> ("NewVal"=w157:bool)  [unwired: 1 in]
        n107 = case shown="True" w157 {
          selector: w157 -> [w161 _]
          tunnel: [w161 w162] -> w159
          frame False {
          }
          frame True {
            n108 = Two Button Dialog(message="Are you sure you want to \"Reset the I/O\"?", 1:"Reset" ("T button name (\"OK\")"), 2:"Return" ("F button name (\"Cancel\")")) -> (T button?=w162:bool)
            n109 = call <vilib>:"Beep.vi"() -> ()  [unwired: 12 in]
          }
        }
        n110 = case shown="False" w159 {
          tunnel: [T9[] [{"Exec States"=enum."HW Close Crtl", "U32"=0, "I32"=0, "DBL_1 (X)"=0.0, "DBL_2 (Y)"=0.0, "DBL_3 (Z)"=0.0, "Bool_1"=FALSE, "Bool_2"=FALSE, "Variant"=variant(string "")}, {"Exec States"=enum."SW Init", "U32"=0, "I32"=0, "DBL_1 (X)"=0.0, "DBL_2 (Y)"=0.0, "DBL_3 (Z)"=0.0, "Bool_1"=FALSE, "Bool_2"=FALSE, "Variant"=variant(string "")}] ("Actions") _] -> w158
          frame False {
            # "0: HW Close Ctrl\n1: SW Init"
          }
          frame True {
          }
        }
      }
      event "Exit": Value Change {
        n111 = event-data() -> ("NewVal"=w170:bool)  [unwired: 1 in]
        n112 = case shown="True" w170 {
          selector: w170 -> [w178 _]
          tunnel: [w178 w179] -> w169
          frame False {
          }
          frame True {
            n113 = Two Button Dialog(message="Are you sure you want to exit the program?", 1:"Quit" ("T button name (\"OK\")"), 2:"Return" ("F button name (\"Cancel\")")) -> (T button?=w179:bool)
          }
        }
        n114 = case shown="False" w169 {
          tunnel: w168 -> [w176 _]
          tunnel: [w175 FALSE ("event data")] -> w166
          tunnel: [w171 _] -> w167
          frame False {
            w175 = TRUE ("event data")
            # "1. Shutdown"
            n115 = Generate User Event(user event=w176, event data cluster=w175) -> ()  [unwired: 2 in, 2 out]
            n116 = Bundle By Name(cluster=T9 {"Exec States"=enum."SW Init", "U32"=0, "I32"=0, "DBL_1 (X)"=0.0, "DBL_2 (Y)"=0.0, "DBL_3 (Z)"=0.0, "Bool_1"=FALSE, "Bool_2"=FALSE, "Variant"=variant(string "")} ("Que"), "Exec States"=Image-DO_with_Stage_-_Exec_States."Shutdown") -> (w173:T9)
            n117 = Build Array(w173) -> (w171:T9[])
          }
          frame True {
          }
        }
      }
      event "Step Mode": Value Change {
        n118 = event-data() -> ("NewVal"=w184:bool)  [unwired: 1 in]
        n119 = property on="Advance" class="Bool (strict)"("Visible"=w184, "DisabledEnum"=2) -> ()  [unwired: 2 in, 2 out]
      }
      event "Amy URL": Mouse Up {
        n120 = event-data() -> ()  [unwired: 1 in, 1 out]
        n121 = call-poly <vilib>:"Open URL in Default Browser.vi"("URL"="https://www.chem.purdue.edu/jafci/index.html") -> ()  [unwired: 5 in, 2 out]
      }
      event "XY Scan Mode": Value Change {
        n122 = event-data() -> ("NewVal"=w186:bool)  [unwired: 1 in]
        n123 = Not(x=w186) -> (.not. x?=w187:bool)
        n124 = property on="User Defined Points" class="Clust (strict)"("Visible"=w186) -> ()  [unwired: 2 in, 2 out]
        n125 = property on="Grid Parameters" class="Clust (strict)"("Visible"=w187) -> ()  [unwired: 2 in, 2 out]
      }
      event Value Change {
        w195 = FALSE ("First")
        n126 = event-data() -> ("OldVal"=w194:T5, "NewVal"=w193:T5)  [unwired: 1 in]
        n127 = Equal?(x=w194, y=w193) -> (x = y?=w192:T18)
        n128 = Unbundle By Name(w192) -> ("First"=w196:bool, "Back"=w197:bool, "Next"=w198:bool, "Last"=w199:bool, "Insert Current"=w200:bool, "Go To"=w201:bool, "Delete"=w202:bool, "Clear"=w203:bool, "Insert"=w204:bool)
        n129 = Build Array(w196, w197, w198, w199, w200, w201, w202, w203, w204) -> (w205:bool[])
        n130 = Search 1D Array(1D array=w205, element=FALSE) -> (index of element=w206:i32)  [unwired: 1 in]
        n131 = case shown="4" w206 {
          tunnel: w193 -> [_ _ _ _ _ _ _ _ w241 _]
          tunnel: [w210 w212 w216 w219 w224 w231 w236 w238 w244 w247] -> w207
          tunnel: [w209 w213 w217 w220 w223 w233 w235 w239 w243 w246] -> w208
          tunnel: [_ _ _ _ _ w225 _ _ _ _] -> w188
          frame 0 {
            # "First"
            n132 = call "Image-DO with Stage - User Defined Pts.vi"("Action"=T14."Go to First") -> ("Status"=w209:string, "Curernt Point"=w210:T6)  [unwired: 7 in, 2 out]
          }
          frame 1 {
            # "Back"
            n133 = call "Image-DO with Stage - User Defined Pts.vi"("Action"=T14."Step Back") -> ("Status"=w213:string, "Curernt Point"=w212:T6)  [unwired: 7 in, 2 out]
          }
          frame 2 {
            # "Next"
            n134 = call "Image-DO with Stage - User Defined Pts.vi"("Action"=T14."Step Forward") -> ("Status"=w217:string, "Curernt Point"=w216:T6)  [unwired: 7 in, 2 out]
          }
          frame 3 {
            # "Last"
            n135 = call "Image-DO with Stage - User Defined Pts.vi"("Action"=T14."Go to Last") -> ("Status"=w220:string, "Curernt Point"=w219:T6)  [unwired: 7 in, 2 out]
          }
          frame 4 {
            # "Insert Current"
            n136 = local read "Current Position"() -> (w221:T6)
            n137 = call "Image-DO with Stage - User Defined Pts.vi"("Action"=T14."Insert", "New Point"=w221) -> ("Status"=w223:string, "Curernt Point"=w224:T6)  [unwired: 6 in, 2 out]
          }
          frame 5 {
            # "Go To"
            n138 = call "Image-DO with Stage - User Defined Pts.vi"("Action"=T14."Read") -> ("Status"=w233:string, "Curernt Point"=w231:T6)  [unwired: 7 in, 2 out]
            n139 = Unbundle By Name(w231) -> ("X Pos"=w229:dbl, "Y Pos"=w228:dbl, "Z Pos"=w227:dbl)
            n140 = Bundle By Name(cluster=T9 {"Exec States"=enum."Set Position - Prior", "U32"=0, "I32"=0, "DBL_1 (X)"=0.0, "DBL_2 (Y)"=0.0, "DBL_3 (Z)"=0.0, "Bool_1"=FALSE, "Bool_2"=FALSE, "Variant"=variant(string "")}, "DBL_1 (X)"=w229, "DBL_2 (Y)"=w228, "DBL_3 (Z)"=w227) -> (w226:T9)
            n141 = Build Array(w226) -> (w225:T9[])
          }
          frame 6 {
            # "Delete"
            n142 = call "Image-DO with Stage - User Defined Pts.vi"("Action"=T14."Delete") -> ("Status"=w235:string, "Curernt Point"=w236:T6)  [unwired: 7 in, 2 out]
          }
          frame 7 {
            # "Clear"
            n143 = call "Image-DO with Stage - User Defined Pts.vi"("Action"=T14."Delete All") -> ("Status"=w239:string, "Curernt Point"=w238:T6)  [unwired: 7 in, 2 out]
          }
          frame 8 {
            # "Insert"
            n144 = Unbundle By Name(w241) -> ("New Position"=w240:T6)
            n145 = call "Image-DO with Stage - User Defined Pts.vi"("Action"=T14."Insert", "New Point"=w240) -> ("Status"=w243:string, "Curernt Point"=w244:T6)  [unwired: 6 in, 2 out]
          }
          frame Default {
            # "No Action"
            n146 = call "Image-DO with Stage - User Defined Pts.vi"("Action"=T14."Read") -> ("Status"=w246:string, "Curernt Point"=w247:T6)  [unwired: 7 in, 2 out]
          }
        }
        n147 = Bundle By Name(cluster="User Defined Points", "Step Position"=w207, "Status"=w208, "First"=w195, "Back"=w195, "Next"=w195, "Last"=w195, "Insert Current"=w195, "Go To"=w195, "Delete"=w195, "Clear"=w195, "Insert"=w195) -> (w190:T5)
        n148 = local write "User Defined Points"(w190) -> ()
      }
      event "Get Masks": Value Change {
        n149 = event-data() -> ("NewVal"=w249:bool)  [unwired: 1 in]
        n150 = case shown="True" w249 {
          tunnel: [_ w250] -> w248
          frame False {
          }
          frame True {
            n151 = Bundle By Name(cluster=T9 {"Exec States"=enum."SW Init", "U32"=0, "I32"=0, "DBL_1 (X)"=0.0, "DBL_2 (Y)"=0.0, "DBL_3 (Z)"=0.0, "Bool_1"=FALSE, "Bool_2"=FALSE, "Variant"=variant(string "")} ("Que"), "Exec States"=Image-DO_with_Stage_-_Exec_States."Pre-Mask Ctrl") -> (w253:T9)
            n152 = Build Array(w253) -> (w250:T9[])
          }
        }
      }
      event "Get Image Mask": Value Change {
        n153 = event-data() -> ("NewVal"=w255:bool)  [unwired: 1 in]
        n154 = case shown="True" w255 {
          tunnel: [_ w257] -> w254
          frame False {
          }
          frame True {
            # "I32: Mask # (-1 Image)\nBool 1 : Common Mask"
            n155 = Bundle By Name(cluster=T9 {"Exec States"=enum."SW Init", "U32"=0, "I32"=0, "DBL_1 (X)"=0.0, "DBL_2 (Y)"=0.0, "DBL_3 (Z)"=0.0, "Bool_1"=FALSE, "Bool_2"=FALSE, "Variant"=variant(string "")} ("Que"), "Exec States"=Image-DO_with_Stage_-_Exec_States."Update Mask", "I32"=-1) -> (w260:T9)
            n156 = Build Array(w260) -> (w257:T9[])
          }
        }
      }
      event "Save Masks": Value Change {
        n157 = event-data() -> ("NewVal"=w262:bool)  [unwired: 1 in]
        n158 = case shown="True" w262 {
          tunnel: [_ w265] -> w261
          frame False {
          }
          frame True {
            # "Save File\n  - Bool1: Append Parameters\n  - Bool2: Mask Save\n        T: Image Mask\n        F: Scan Masks\n  - Variant: File Operation"
            n159 = Bundle By Name(cluster=T9 {"Exec States"=enum."SW Init", "U32"=0, "I32"=0, "DBL_1 (X)"=0.0, "DBL_2 (Y)"=0.0, "DBL_3 (Z)"=0.0, "Bool_1"=FALSE, "Bool_2"=FALSE, "Variant"=variant(string "")} ("Que"), "Exec States"=Image-DO_with_Stage_-_Exec_States."Save Files", "Variant"=Image-DO_with_Stage_-_File_Save_Option."Save Mask" ("Action"), "Bool_2"=FALSE) -> (w268:T9)
            n160 = Build Array(w268) -> (w265:T9[])
          }
        }
      }
      event "Common Mask": Value Change {
        n161 = event-data() -> ("NewVal"=w270:bool)  [unwired: 1 in]
        n162 = Select(t=2, s=w270, f=0) -> (s? t:f=w269:i32)
        n163 = property on="Get Masks" class="Bool (strict)"("DisabledEnum"=w269) -> ()  [unwired: 2 in, 2 out]
        n164 = property on="Save Masks" class="Bool"("DisabledEnum"=w269) -> ()  [unwired: 2 in, 2 out]
      }
    }
    n165 = call "Image-DO with Stage - Que Actions.vi"("Actions"=w22, "Qqu Ref In"=w21) -> ("error out"=w20:errorcluster)  [unwired: 8 in, 1 out]
  }
  n166 = while {
    shift-right: [w289] -> _
    shift-left: w11 -> [w291]
    tunnel: w10 -> [w285]
    shift-right: [w283] -> _
    shift-left: _ -> [w284]
    tunnel: [w281] -> w8
    shift-right: [w279] -> _
    shift-left: _ -> [w280]
    stop <- w282 stop-if-true
    # "VISA"
    # "Current Images"
    n167 = Preview Queue Element(queue=w285) -> (queue out=w290:refnum<queue>, element=w287:T9)  [unwired: 2 in, 2 out]
    n168 = disable-structure shown="Default" {
      disable-tunnel: [w297 w303] -> w278
      disable-tunnel: [w296 w302] -> w277
      disable-tunnel: [w295 w301] -> w276
      disable-tunnel: [w294 w300] -> w275
      disable-tunnel: [w293 w299] -> w274
      disable-tunnel: [w292 w298] -> w273
      frame condition #0 {
        w292 = TRUE  # RunTime
        w293 = FALSE  # Reserve 1
        w294 = FALSE  # Zaber
        w295 = FALSE  # Prior
        w296 = FALSE  # DAQmx
        w297 = FALSE  # Reserve 2
      }
      frame condition #1 (active) {
        w298 = FALSE  # RunTime
        w299 = FALSE  # Reserve 1
        w300 = FALSE  # Zaber
        w301 = FALSE  # Prior
        w302 = FALSE  # DAQmx
        w303 = FALSE  # Reserve 2
      }
    }
    n169 = Unbundle By Name(w287) -> ("Exec States"=w286:T10)
    n170 = case shown="\"Mask Crtl\"" w286 {
      tunnel: [w329 w353 w361 w381 w399 w400 w414 w461 w475 w485 w502 w548 w573 w587 w606 w615 w637 w651 w683 w694 w738 w739 w753 w774 w781 w820 w835 w857 w876 w920 w947 w960 w984 w990 w1020 w1025 w1035 w1041 w1046 w1058 w1089 w1112 w1142 w1147 w1151 w1173 w1178 w1212 w1224 w1230 w1231 w1239 w1252 w1256 w1268 errorcluster {"status"=FALSE, "code"=0, "source"=""} ("error out") w1298] -> w289
      tunnel: w291 -> [w316 w353 w371 w382 w399 w400 w414 w462 w475 w485 w502 w548 w574 w587 w606 w615 w636 w651 w683 w694 w738 w740 w753 w774 w781 w821 w835 w857 w876 w920 w946 w960 w984 w990 w1021 w1026 w1034 w1040 w1047 w1059 w1090 w1113 w1142 w1147 w1151 w1174 w1179 w1213 w1224 w1230 w1234 w1240 w1252 w1256 w1268 w1275 w1298]
      tunnel: [w336 w350 w372 w387 w396 w403 w411 w465 w472 w487 w499 w545 w578 w584 w608 w610 w641 w650 w682 w689 w733 w744 w752 w773 w778 w825 w832 w860 w874 w917 w951 w957 w985 w991 w1022 w1029 w1037 w1045 w1048 w1060 w1091 w1118 w1143 w1145 w1149 w1176 w1193 w1217 w1223 w1227 w1237 w1243 w1251 w1254 w1265 w1277 w1303] -> w288
      tunnel: w290 -> [w336 w351 w372 w387 w396 w403 w412 w465 w472 w487 w498 w546 w578 w584 w608 w611 w641 w650 w682 w690 w734 w744 w752 w773 w779 w825 w832 w860 w873 w918 w951 w957 w985 w991 w1022 w1029 w1037 w1045 w1048 w1060 w1091 w1118 w1143 w1145 w1149 w1176 w1193 w1217 w1223 w1228 w1237 w1243 w1251 w1254 w1266 w1280 w1303]
      tunnel: w287 -> [_ _ _ _ _ _ _ _ _ _ w496 _ _ _ _ _ _ _ _ w691 _ _ _ _ _ _ _ _ w871 _ _ _ _ w989 w1016 _ w1036 w1042 _ w1055 w1088 w1115 _ _ _ w1175 w1180 w1214 _ _ _ _ _ _ _ _ _]
      tunnel: w284 -> [_ w352 w373 w388 w397 w402 w413 w464 w473 w480 w500 w547 w577 w585 w603 w614 w640 w649 w681 w693 w737 w743 w751 w772 w780 w824 w833 w854 w875 w919 w950 w958 w982 w987 w1023 w1028 _ w1044 w1049 w1061 w1092 w1117 w1140 w1144 w1148 w1162 w1192 w1216 w1222 w1229 w1236 w1242 w1250 w1255 w1267 w1276 w1302]
      tunnel: [dbl[][][] [] w352 w373 w388 w397 w402 w413 w464 w473 w480 w500 w547 w577 w585 w603 w614 w640 w649 w681 w693 w737 w743 w751 w772 w780 w824 w833 w854 w875 w919 w950 w958 w982 w987 w1023 w1028 w1033 w1044 w1049 w1061 w1092 w1117 w1140 w1144 w1148 w1162 w1192 w1216 w1222 w1229 w1236 w1242 w1250 w1255 w1267 w1276 w1302] -> w283
      tunnel: [_ _ _ _ _ _ _ _ _ _ _ _ _ _ _ _ _ _ _ _ _ _ _ _ _ _ _ _ _ _ _ _ _ _ _ _ _ _ _ _ _ _ _ _ _ _ _ _ _ _ _ _ _ _ _ _ TRUE] -> w282
      tunnel: w280 -> [_ w349 w374 w389 w398 w401 w410 w463 w474 w486 w501 w544 w576 w586 w607 w613 w639 w648 w680 w692 w736 w742 w750 w771 w777 w823 w834 w859 w872 w916 w949 w959 w983 w986 w1024 w1027 w1038 w1043 w1050 w1062 w1093 w1116 w1141 w1146 w1150 w1177 w1191 w1215 w1221 w1225 w1235 w1241 w1249 w1253 w1263 w1271 w1300]
      tunnel: [w332 w349 w374 w389 w398 w401 w410 w463 w474 w486 w501 w544 w576 w586 w607 w613 w639 w648 w680 w692 w736 w742 w750 w771 w777 w823 w834 w859 w872 w916 w949 w959 w983 w986 w1024 w1027 w1038 w1043 w1050 w1062 w1093 w1116 w1141 w1146 w1150 w1177 w1191 w1215 w1221 w1225 w1235 w1241 w1249 w1253 w1263 w1271 w1300] -> w279
      tunnel: w278 -> [_ _ _ _ _ _ _ _ _ _ _ _ _ _ _ _ _ _ _ _ _ _ _ _ _ _ _ _ _ _ _ _ _ _ _ _ _ _ _ _ _ _ _ _ _ _ _ _ _ _ _ _ _ _ _ _ _]
      tunnel: w277 -> [_ _ _ _ _ _ _ _ _ _ _ _ _ _ _ _ _ _ _ _ _ _ _ _ _ _ _ _ _ _ _ _ _ _ _ _ _ _ _ _ _ _ _ _ _ _ _ _ _ _ _ _ _ _ _ _ _]
      tunnel: w276 -> [_ _ _ w380 _ _ _ _ _ _ _ _ _ _ _ _ _ _ _ _ _ _ _ _ _ _ _ _ _ _ _ _ _ _ _ _ _ _ _ w1057 w1086 w1111 _ _ _ _ _ _ _ _ _ w1238 _ _ _ _ _]
      tunnel: w275 -> [_ _ _ _ _ _ _ _ _ _ _ _ _ _ _ _ _ _ _ _ _ _ _ _ _ _ _ _ _ _ _ _ _ _ _ _ _ _ _ _ _ _ _ _ _ _ _ _ _ _ _ _ _ _ _ _ _]
      tunnel: w274 -> [_ _ _ _ _ _ _ _ _ _ _ _ _ _ _ _ _ _ _ _ _ _ _ _ _ _ _ _ _ _ _ _ _ _ _ _ _ _ _ _ _ _ _ _ _ _ _ _ _ _ _ _ _ _ _ _ _]
      tunnel: w273 -> [_ _ _ _ _ _ _ _ _ _ _ _ _ _ _ _ _ _ _ _ _ _ _ _ _ _ _ _ _ _ _ _ _ _ _ _ _ _ _ _ _ _ _ _ _ _ _ _ _ _ _ _ _ _ _ _ w1295]
      frame "SW Init" {
        w327 = FALSE ("Visible")
        w320 = FALSE ("Auto Save")
        w326 = 2
        w332 = refnum<visa-resource-name> refnum  # VISA resource
        w324 = u8 0 ("Disabled")
        w325 = FALSE ("Scan")
        # "Data Structure\nMask #\nMask Y Data\nMask X Data"
        # "Data Structure\nImage #\nImage Y Data\nImage X Data"
        n171 = property on="Path" class="Path"("DisabledEnum"=w324) -> ()  [unwired: 2 in, 2 out]
        n172 = property on="Base Filename" class="Str"("DisabledEnum"=w324) -> ()  [unwired: 2 in, 2 out]
        n173 = property on="Get Image Mask" class="Bool"("DisabledEnum"=w324) -> ()  [unwired: 2 in, 2 out]
        n174 = property on="Get Masks" class="Bool (strict)"("DisabledEnum"=w324, "Blinking"=FALSE) -> ()  [unwired: 2 in, 2 out]
        n175 = property on="Reset I/O" class="Bool"("Disabled"=w324) -> ()  [unwired: 2 in, 2 out]
        n176 = property on="Exit" class="Bool"("Disabled"=w324) -> ()  [unwired: 2 in, 2 out]
        n177 = property on="Operation" class="TabCtl (strict)"("Disabled"=w324) -> ()  [unwired: 2 in, 2 out]
        n178 = property on="Aquire Image" class="Bool (strict)"("DisabledEnum"=w324, "Blinking"=w325, "Value"=w325) -> ()  [unwired: 2 in, 2 out]
        n179 = property on="Connect" class="Bool (strict)"("Disabled"=w324, "Blinking"=w325, "Value"=w325) -> ()  [unwired: 2 in, 2 out]
        n180 = property on="Scan" class="Bool (strict)"("DisabledEnum"=w324, "Blinking"=w325, "Value"=w325) -> ()  [unwired: 2 in, 2 out]
        n181 = property on="Aquire Image" class="Bool (strict)"("DisabledEnum"=w324, "Blinking"=w325, "Value"=w325) -> ()  [unwired: 2 in, 2 out]
        n182 = property on="Main Tab" class="TabCtl (strict)"("Value"=enum32{"I/O Config", "Image"}."I/O Config" ("Main Tab"), "Tabs Visible?"=FALSE) -> ()  [unwired: 2 in, 2 out]
        n183 = property on="Save Image" class="Bool"("Disabled"=w326) -> ()  [unwired: 2 in, 2 out]
        n184 = property on="Advance" class="Bool (strict)"("DisabledEnum"=w326, "Visible"=w327, "Blinking"=w327) -> ()  [unwired: 2 in, 2 out]
        n185 = Current VI's Path() -> (path=w318:path)
        n186 = call "Set Pannel Size..vi"("error in (no error)"=w316, "FP:Window Bounds"=T20 {"Left"=0, "Top"=0, "Right"=2480, "Bottom"=1480}, "VI path"=w318) -> ("error out"=w315:errorcluster)  [unwired: 8 in]
        n187 = call "Image-DO with Stage - System State.vi"("Set State (F:Get)"=TRUE ("Action (F:Get)"), "Sys State In"=Image-DO_with_Stage_-_Sys_State."HW Un_init") -> ()  [unwired: 7 in, 3 out]
        n188 = First Call?() -> (First Call?: T/F=w330:bool)
        n189 = case shown="True" w330 {
          tunnel: [w337 w341] -> w329
          tunnel: w315 -> [w337 w338]
          frame False {
          }
          frame True {
            # "This does not get reloaded durteting a channel reset"
            n190 = call "Get path to Image Display Sub Pannel.vi"("error in (no error)"=w338) -> ("error out"=w339:errorcluster, "Sup Pannel VI Path"=w340:path)  [unwired: 9 in]
            n191 = Open VI Reference(vi path=w340, error in (no error)=w339) -> (vi reference=w345:refnum<vi>, error out=w344:errorcluster)  [unwired: 4 in]
            n192 = invoke class="VI" method="Run VI"(reference=w345, error in=w344, "Wait until done"=FALSE ("Wait Until Done"), "Auto Dispose Ref"=FALSE ("Auto Dispose Reference")) -> (reference out=w342:refnum<vi>, error out=w343:errorcluster)  [unwired: 1 in, 3 out]
            n193 = invoke on="Display" class="SubPnl" method="Insert VI"(error in=w343, "VI Ref"=w342) -> (error out=w341:errorcluster)  [unwired: 2 in, 3 out]
          }
        }
        n194 = local read "Imageing Parameters"() -> (w312:T2)
        n195 = call "Image-DO with Stage - DO Masks.vi"("Action"=T19."Set Imaging Mask", "Image Mask"=u8[][] []) -> ()  [unwired: 8 in, 2 out]
        n196 = local read "XY Scan Mode"() -> (w310:bool)
        n197 = Unbundle By Name(w312) -> ("Sample Rate"=w311:dbl)
        n198 = property on="Sample Rate" class="DigNum (strict)"("Val(Sgnl)"=w311) -> ()  [unwired: 2 in, 2 out]
        n199 = property on="XY Scan Mode" class="Bool (strict)"("Val(Sgnl)"=w310) -> ()  [unwired: 2 in, 2 out]
        n200 = call "Image-DO with Stage - DO Masks.vi"("Action"=T19."Set Scan Masks", "Scan Masks In"=u8[][][] []) -> ()  [unwired: 8 in, 2 out]
        n201 = local write "Status"("Ready" ("Status")) -> ()
        n202 = local write "Auto Save"(w320) -> ()
        n203 = local write "Step Mode"(w320) -> ()
        n204 = local write "Common Mask"(w320) -> ()
      }
      frame "HW Init Ctrl" {
        # "0: HW Init - DAQmx\n1: HW Init - Prior\n2: HW Init - SW"
        n205 = call "Image-DO with Stage - Que Actions.vi"("Actions"=T9[] [{"Exec States"=enum."HW Init - DAQmx", "U32"=0, "I32"=0, "DBL_1 (X)"=0.0, "DBL_2 (Y)"=0.0, "DBL_3 (Z)"=0.0, "Bool_1"=FALSE, "Bool_2"=FALSE, "Variant"=variant(string "")}, {"Exec States"=enum."HW Init - Prior", "U32"=0, "I32"=0, "DBL_1 (X)"=0.0, "DBL_2 (Y)"=0.0, "DBL_3 (Z)"=0.0, "Bool_1"=FALSE, "Bool_2"=FALSE, "Variant"=variant(string "")}, {"Exec States"=enum."HW Init - SW", "U32"=0, "I32"=0, "DBL_1 (X)"=0.0, "DBL_2 (Y)"=0.0, "DBL_3 (Z)"=0.0, "Bool_1"=FALSE, "Bool_2"=FALSE, "Variant"=variant(string "")}], "Qqu Ref In"=w351) -> ("Que Ref Out"=w350:refnum<queue>)  [unwired: 8 in, 1 out]
      }
      frame "HW Init - DAQmx" {
        n206 = call "Imager - Create DAQmx AO Task.vi"("error in (no error)"=w371, "Y-Mirror DAQmx AO Channel"="Y-Mirror DAQmx AO Channel", "X-Mirror DAQmx AO Channel"="X-Mirror DAQmx AO Channel") -> ("error out"=w368:errorcluster)  [unwired: 8 in]
        n207 = call "Imager - Create DAQmx AI Task.vi"("Max Input Value (1)"="Max Value", "Min Input Value (0)"="Min Value", "error in (no error)"=w368, "DAQmx AI Channels"="DAQmx AI Channels") -> ("error out"=w367:errorcluster)  [unwired: 7 in]
        n208 = call "Imager - Create DAQmx DO Task.vi"("error in (no error)"=w367, "DAQmx DO Port"="DAQmx DO Port") -> ("error out"=w362:errorcluster)  [unwired: 9 in]
        n209 = Not Equal?(x=tag "" ("DAQmx Static DO Lines"), y="DAQmx Static DO Lines") -> (x != y?=w356:bool)
        n210 = case shown="True" w356 {
          tunnel: w362 -> [w375 w379]
          tunnel: [w375 w378] -> w361
          tunnel: "DAQmx Static DO Lines" -> [_ w376]
          frame False {
          }
          frame True {
            n211 = call "Image-DO with Stage - Set Static DO.vi"("Action"=T21."Create Task", "error in"=w379, "DAQmx Lines"=w376) -> ("error out"=w378:errorcluster)  [unwired: 8 in]
          }
        }
        n212 = Select(t=0, s=w356, f=2) -> (s? t:f=w355:i32)
        n213 = property on="Statice DO" class="Arr (strict)"("DisabledEnum"=w355, "Value"=bool[] [FALSE, FALSE, FALSE, FALSE, FALSE, FALSE, FALSE, FALSE]) -> ()  [unwired: 2 in, 2 out]
      }
      frame "HW Init - Prior" {
        n214 = Scan From String(format string="COM%d", input string="Prior Stage VISA Resource", default 1=0 ("default value 1")) -> (output 1=w383:i32)  [unwired: 2 in, 3 out]
        n215 = case shown="False" w380 {
          tunnel: w383 -> [w394 _]
          tunnel: w382 -> [w391 w395]
          tunnel: [w390 w395] -> w381
          frame False {
            n216 = call "IScan Open.vi"("error in (no error)"=w391, "Port"=w394) -> ("error out"=w393:errorcluster)  [unwired: 2 in, 1 out]
            n217 = call "IStage Open.vi"("error in (no error)"=w393) -> ("error out"=w392:errorcluster)  [unwired: 2 in]
            n218 = call "IZ Open.vi"("error in (no error)"=w392) -> ("error out"=w390:errorcluster)  [unwired: 2 in]
          }
          frame True {
          }
        }
      }
      frame "HW Init - Reserve 1", "HW Init - Reserve 2" {
        # "Place Holder"
      }
      frame "HW Init - SW" {
        n219 = stacked-sequence {
          frame #0 {
            w404 = FALSE ("Scan")
            # "Enable/Disable FP Contols"
            n220 = property on="Connect" class="Bool (strict)"("Blinking"=w404, "Value"=w404) -> ()  [unwired: 2 in, 2 out]
          }
          frame #1 {
            # "Show Pages"
            n221 = property on="Main Tab" class="TabCtl (strict)"("Value"=enum32{"I/O Config", "Image"}."Image" ("Main Tab")) -> ()  [unwired: 2 in, 2 out]
          }
          frame #2 {
            # "Update DAQ system state/status"
            n222 = call "Image-DO with Stage - System State.vi"("Set State (F:Get)"=TRUE ("Action (F:Get)"), "Sys State In"=Image-DO_with_Stage_-_Sys_State."HW Initialized") -> ()  [unwired: 7 in, 3 out]
          }
        }
      }
      frame "Pre-Image Crtl" {
        # "- DAQmx\n  - I32: Mask Index\n  - Bool 1\n        T: Continuous Mode\n         F: Finite Mode\n\nSave File\n  - Bool1: Append Parameters\n  - Bool2: Mask Save\n        T: Image Mask\n        F: Scan Masks\n  - Variant: File Operation"
        # "0: Configure Imaging - DAQmx (BL1: F ,I32:-1)\n1: Pre-Image - DAQmx  \n2: Pre-Image - Prior\n3: Pre-Image - SW\n4: Save Parameter File  / Wait (BL1: F, BL2: T))\n5: Open Data Files\n6: Image Ctrl (Bool 1,T)"
        n223 = for {
          N: 7 -> [_]
          tunnel: [w415] -> w408 mode=indexing
          i -> [w416]
          n224 = case shown="0" w416 {
            tunnel: T9 {"Exec States"=enum."SW Init", "U32"=0, "I32"=0, "DBL_1 (X)"=0.0, "DBL_2 (Y)"=0.0, "DBL_3 (Z)"=0.0, "Bool_1"=FALSE, "Bool_2"=FALSE, "Variant"=variant(string "")} ("Que") -> [w422 w425 w428 w431 w436 w446 w455 w458]
            tunnel: [w421 w424 w427 w430 w435 w445 w454 w457] -> w415
            frame 0 {
              n225 = Bundle By Name(cluster=w422, "Exec States"=Image-DO_with_Stage_-_Exec_States."Confgure Imaging - DAQmx", "Bool_1"=FALSE, "I32"=-1) -> (w421:T9)
            }
            frame 1 {
              n226 = Bundle By Name(cluster=w425, "Exec States"=Image-DO_with_Stage_-_Exec_States."Pre-Image HW - DAQmx") -> (w424:T9)
            }
            frame 2 {
              n227 = Bundle By Name(cluster=w428, "Exec States"=Image-DO_with_Stage_-_Exec_States."Pre-Image HW - Prior") -> (w427:T9)
            }
            frame 3 {
              n228 = Bundle By Name(cluster=w431, "Exec States"=Image-DO_with_Stage_-_Exec_States."Pre-Image SW") -> (w430:T9)
            }
            frame 4 {
              n229 = local read "Auto Save"() -> (w441:bool)
              n230 = Select(t=Image-DO_with_Stage_-_Exec_States."Save Files" ("Exec States"), s=w441, f=Image-DO_with_Stage_-_Exec_States."Wait (ms)" ("Exec States")) -> (s? t:f=w440:T10)
              n231 = To Variant(anything=Image-DO_with_Stage_-_File_Save_Option."Save Image Parameters" ("Action")) -> (Variant=w439:variant)
              n232 = Bundle By Name(cluster=w436, "Exec States"=w440, "Variant"=w439, "Bool_1"=FALSE, "Bool_2"=TRUE) -> (w435:T9)
            }
            frame 5 {
              n233 = local read "Auto Save"() -> (w451:bool)
              n234 = Select(t=Image-DO_with_Stage_-_Exec_States."Save Files" ("Exec States"), s=w451, f=Image-DO_with_Stage_-_Exec_States."Wait (ms)" ("Exec States")) -> (s? t:f=w450:T10)
              n235 = To Variant(anything=Image-DO_with_Stage_-_File_Save_Option."Open Data Files" ("Action")) -> (Variant=w449:variant)
              n236 = Bundle By Name(cluster=w446, "Exec States"=w450, "Variant"=w449, "Bool_1"=TRUE, "Bool_2"=FALSE) -> (w445:T9)
            }
            frame 6 {
              n237 = Bundle By Name(cluster=w455, "Exec States"=Image-DO_with_Stage_-_Exec_States."Image Ctrl", "Bool_1"=TRUE) -> (w454:T9)
            }
            frame Default {
              # "Invalid case"
              n238 = Bundle By Name(cluster=w458, "Exec States"=Image-DO_with_Stage_-_Exec_States."Wait (ms)") -> (w457:T9)
            }
          }
        }
        n239 = call "Image-DO with Stage - Que Actions.vi"("Actions"=w408, "Qqu Ref In"=w412) -> ("Que Ref Out"=w411:refnum<queue>)  [unwired: 8 in, 1 out]
      }
      frame "Pre-Image HW - DAQmx" {
        n240 = property on="Statice DO" class="Arr (strict)"() -> ("Visible"=w460:bool, "Value"=w459:bool[])  [unwired: 2 in, 2 out]
        n241 = case shown="True" w460 {
          tunnel: w462 -> [w466 w470]
          tunnel: [w466 w469] -> w461
          tunnel: w459 -> [_ w468]
          frame False {
          }
          frame True {
            n242 = Boolean Array To Number(Boolean array=w468) -> (number=w467:u32)
            n243 = call "Image-DO with Stage - Set Static DO.vi"("Action"=T21."Write Lnes", "error in"=w470, "line data"=w467) -> ("error out"=w469:errorcluster)  [unwired: 8 in]
          }
        }
      }
      frame "Pre-Image HW - Prior".."Pre-Image HW - Reserve 2" {
        # "Place Holder"
      }
      frame "Pre-Image SW" {
        w476 = u8 2 ("Disabled")
        # "Pre-configure the data space and GUI for data acquisition."
        n244 = call "Image-DO with Stage - System State.vi"("Set State (F:Get)"=TRUE ("Action (F:Get)"), "Sys State In"=Image-DO_with_Stage_-_Sys_State."Imaging") -> ()  [unwired: 7 in, 3 out]
        n245 = local write "Status"("** Starting Image Scan **" ("Status")) -> ()
        n246 = call "Image-DO with Stage - User GUI Settings.vi"("Action (0: Read All)"=T11."Set Descriptor", "File Descriptor In"="") -> ()  [unwired: 8 in, 6 out]
        n247 = property on="Exit" class="Bool"("Disabled"=w476) -> ()  [unwired: 2 in, 2 out]
        n248 = property on="Get Image Mask" class="Bool"("DisabledEnum"=w476) -> ()  [unwired: 2 in, 2 out]
        n249 = property on="Get Masks" class="Bool (strict)"("DisabledEnum"=w476) -> ()  [unwired: 2 in, 2 out]
        n250 = property on="Save Masks" class="Bool"("DisabledEnum"=w476) -> ()  [unwired: 2 in, 2 out]
        n251 = property on="Common Mask" class="Bool (strict)"("DisabledEnum"=w476) -> ()  [unwired: 2 in, 2 out]
        n252 = property on="Scan" class="Bool (strict)"("DisabledEnum"=w476) -> ()  [unwired: 2 in, 2 out]
        n253 = property on="Save Image" class="Bool"("DisabledEnum"=w476) -> ()  [unwired: 2 in, 2 out]
        n254 = property on="Reset I/O" class="Bool"("DisabledEnum"=w476) -> ()  [unwired: 2 in, 2 out]
        n255 = property on="Operation" class="TabCtl (strict)"("DisabledEnum"=w476, "Value"=enum32{"Imaging", "Stage Scan"}."Imaging" ("Operation")) -> ()  [unwired: 2 in, 2 out]
        n256 = property on="Aquire Image" class="Bool (strict)"("Blinking"=TRUE) -> ()  [unwired: 2 in, 2 out]
      }
      frame "Image Ctrl" {
        # "Configure Imaging - DAQmx\n  - I32: Mask Index\n  - Bool 1\n        T: Continuous Mode\n         F: Finite Mode\n\nSave File\n  - Bool1: Append Parameters\n  - Bool2: Mask Save\n        T: Image Mask\n        F: Scan Masks\n  - Variant: File Operation"
        # "First Call"
        n257 = Unbundle By Name(w496) -> ("Bool_1"=w494:bool)
        n258 = feedback #1() -> (w492:i32)  [unwired: 1 in]
        n259 = Select(t=0, s=w494, f=w492) -> (s? t:f=w493:i32)
        n260 = Increment(x=w493) -> (x+1=w490:i32)
        n261 = feedback-in #1(w490) -> ()
        n262 = Format Into String(format string="** Imaging **\nCollecting Image %d", w490) -> (resulting string=w488:string)  [unwired: 2 in, 1 out]
        n263 = local write "Status"(w488) -> ()
        n264 = case shown="True" "Aquire Image" {
          tunnel: [w504 T9[] [{"Exec States"=enum."Post-Image Crtl", "U32"=0, "I32"=0, "DBL_1 (X)"=0.0, "DBL_2 (Y)"=0.0, "DBL_3 (Z)"=0.0, "Bool_1"=FALSE, "Bool_2"=FALSE, "Variant"=variant(string "")}] ("Actions")] -> w497
          frame True {
            # "0: Start Imaging\n1: ReadImages (DBL_1: 60)\n2: Stop Imaging\n3: Process Data\n4: Display Image\n5: Save Scan / Wait ms\n6: Image Ctrl"
            # "Keep imaging"
            n265 = for {
              N: 7 -> [_]
              tunnel: [w505] -> w504 mode=indexing
              i -> [w506]
              n266 = case shown="5" w506 {
                tunnel: T9 {"Exec States"=enum."SW Init", "U32"=0, "I32"=0, "DBL_1 (X)"=0.0, "DBL_2 (Y)"=0.0, "DBL_3 (Z)"=0.0, "Bool_1"=FALSE, "Bool_2"=FALSE, "Variant"=variant(string "")} ("Que") -> [w511 w515 w518 w521 w524 w529 w537 w540]
                tunnel: [w510 w514 w517 w520 w523 w528 w536 w539] -> w505
                frame 0 {
                  n267 = Bundle By Name(cluster=w511, "Exec States"=Image-DO_with_Stage_-_Exec_States."Start Imaging - DAQmx", "DBL_1 (X)"=60.0) -> (w510:T9)
                }
                frame 1 {
                  n268 = Bundle By Name(cluster=w515, "Exec States"=Image-DO_with_Stage_-_Exec_States."Read Images - DAQmx", "DBL_1 (X)"=60.0) -> (w514:T9)
                }
                frame 2 {
                  n269 = Bundle By Name(cluster=w518, "Exec States"=Image-DO_with_Stage_-_Exec_States."Stop Imaging - DAQmx") -> (w517:T9)
                }
                frame 3 {
                  n270 = Bundle By Name(cluster=w521, "Exec States"=Image-DO_with_Stage_-_Exec_States."Process Data") -> (w520:T9)
                }
                frame 4 {
                  n271 = Bundle By Name(cluster=w524, "Exec States"=Image-DO_with_Stage_-_Exec_States."Display Image") -> (w523:T9)
                }
                frame 5 {
                  n272 = local read "Auto Save"() -> (w534:bool)
                  n273 = Select(t=Image-DO_with_Stage_-_Exec_States."Save Files" ("Exec States"), s=w534, f=Image-DO_with_Stage_-_Exec_States."Wait (ms)" ("Exec States")) -> (s? t:f=w533:T10)
                  n274 = To Variant(anything=Image-DO_with_Stage_-_File_Save_Option."Append Data Files" ("Action")) -> (Variant=w532:variant)
                  n275 = Bundle By Name(cluster=w529, "Exec States"=w533, "Variant"=w532, "Bool_1"=FALSE, "Bool_2"=TRUE) -> (w528:T9)
                }
                frame 6 {
                  n276 = Bundle By Name(cluster=w537, "Exec States"=Image-DO_with_Stage_-_Exec_States."Image Ctrl") -> (w536:T9)
                }
                frame Default {
                  # "Invalid case"
                  n277 = Bundle By Name(cluster=w540, "Exec States"=Image-DO_with_Stage_-_Exec_States."Wait (ms)") -> (w539:T9)
                }
              }
            }
          }
          frame False {
            # "Stop imaging"
            # "0: Post Image Ctrl"
          }
        }
        n278 = call "Image-DO with Stage - Que Actions.vi"("Actions"=w497, "Qqu Ref In"=w498) -> ("Que Ref Out"=w499:refnum<queue>)  [unwired: 8 in, 1 out]
      }
      frame "Post-Image Crtl" {
        # "Configure Imaging - DAQmx\n  - I32: Mask Index\n  - Bool 1\n        T: Continuous Mode\n         F: Finite Mode\n\nSave File\n  - Bool1: Append Parameters\n  - Bool2: Mask Save\n        T: Image Mask\n        F: Scan Masks\n  - Variant: File Operation"
        # "Keep imaging"
        # "0: Post-Image - DAQmx\n1: Post-Image - Prior\n2: Post-Image - SW\n3: Close Files (Bl1: T)"
        n279 = for {
          N: 4 -> [_]
          tunnel: [w549] -> w542 mode=indexing
          i -> [w550]
          n280 = case shown="3" w550 {
            tunnel: T9 {"Exec States"=enum."SW Init", "U32"=0, "I32"=0, "DBL_1 (X)"=0.0, "DBL_2 (Y)"=0.0, "DBL_3 (Z)"=0.0, "Bool_1"=FALSE, "Bool_2"=FALSE, "Variant"=variant(string "")} ("Que") -> [w554 w557 w560 w564 w572]
            tunnel: [w553 w556 w559 w563 w571] -> w549
            frame 0 {
              n281 = Bundle By Name(cluster=w554, "Exec States"=Image-DO_with_Stage_-_Exec_States."Post-Image HW - DAQmx") -> (w553:T9)
            }
            frame 1 {
              n282 = Bundle By Name(cluster=w557, "Exec States"=Image-DO_with_Stage_-_Exec_States."Post-Image HW - Prior") -> (w556:T9)
            }
            frame 2 {
              n283 = Bundle By Name(cluster=w560, "Exec States"=Image-DO_with_Stage_-_Exec_States."Post-Image SW") -> (w559:T9)
            }
            frame 3 {
              n284 = local read "Auto Save"() -> (w569:bool)
              n285 = Select(t=Image-DO_with_Stage_-_Exec_States."Save Files" ("Exec States"), s=w569, f=Image-DO_with_Stage_-_Exec_States."Wait (ms)" ("Exec States")) -> (s? t:f=w568:T10)
              n286 = To Variant(anything=Image-DO_with_Stage_-_File_Save_Option."Close Data Files" ("Action")) -> (Variant=w567:variant)
              n287 = Bundle By Name(cluster=w564, "Exec States"=w568, "Variant"=w567, "Bool_1"=TRUE) -> (w563:T9)
            }
            frame Default {
              # "Invalid case"
              n288 = Bundle By Name(cluster=w572, "Exec States"=Image-DO_with_Stage_-_Exec_States."Wait (ms)") -> (w571:T9)
            }
          }
        }
        n289 = call "Image-DO with Stage - Que Actions.vi"("Actions"=w542, "Qqu Ref In"=w546) -> ("Que Ref Out"=w545:refnum<queue>)  [unwired: 8 in, 1 out]
      }
      frame "Post-Image HW - DAQmx" {
        n290 = property on="Statice DO" class="Arr (strict)"() -> ("Visible"=w575:bool)  [unwired: 2 in, 2 out]
        n291 = case shown="True" w575 {
          tunnel: w574 -> [w579 w581]
          tunnel: [w579 w580] -> w573
          frame False {
          }
          frame True {
            n292 = call "Image-DO with Stage - Set Static DO.vi"("Action"=T21."Write Lnes", "error in"=w581, "line data"=u8 0) -> ("error out"=w580:errorcluster)  [unwired: 8 in]
          }
        }
      }
      frame "Post-Image HW - Prior".."Post-Image HW - Reserve 2" {
        # "Place Holder"
      }
      frame "Post-Image SW" {
        w599 = FALSE ("Blinking")
        w600 = u8 0 ("Disabled")
        # "Pre-configure the data space and GUI for POST data acquisition."
        n293 = local read "Status"() -> (w589:string)
        n294 = Scan From String(format string="%d", input string=w589, initial scan location=u32 30, default 1=0 ("default value 1")) -> (output 1=w594:i32)  [unwired: 1 in, 3 out]
        n295 = call "Image-DO with Stage - User GUI Settings.vi"("Action (0: Read All)"=T11."Set Descriptor", "File Descriptor In"="") -> ()  [unwired: 8 in, 6 out]
        n296 = call "Image-DO with Stage - System State.vi"("Set State (F:Get)"=TRUE ("Action (F:Get)"), "Sys State In"=Image-DO_with_Stage_-_Sys_State."Configured") -> ()  [unwired: 7 in, 3 out]
        n297 = Format Into String(format string="** Imaging stopped **\n%d images aquired" ("Status"), w594) -> (resulting string=w588:string)  [unwired: 2 in, 1 out]
        n298 = local write "Status"(w588) -> ()
        n299 = property on="Aquire Image" class="Bool (strict)"("Blinking"=w599, "Value"=w599) -> ()  [unwired: 2 in, 2 out]
        n300 = local read "Common Mask"() -> (w598:bool)
        n301 = Select(t=u8 2 ("Disabled"), s=w598, f=u8 0) -> (s? t:f=w596:u8)
        n302 = property on="Exit" class="Bool"("Disabled"=w600) -> ()  [unwired: 2 in, 2 out]
        n303 = property on="Get Image Mask" class="Bool"("DisabledEnum"=w600) -> ()  [unwired: 2 in, 2 out]
        n304 = property on="Common Mask" class="Bool (strict)"("DisabledEnum"=w600) -> ()  [unwired: 2 in, 2 out]
        n305 = property on="Scan" class="Bool (strict)"("DisabledEnum"=w600) -> ()  [unwired: 2 in, 2 out]
        n306 = property on="Save Image" class="Bool"("DisabledEnum"=w600) -> ()  [unwired: 2 in, 2 out]
        n307 = property on="Reset I/O" class="Bool"("DisabledEnum"=w600) -> ()  [unwired: 2 in, 2 out]
        n308 = property on="Auto Save" class="Bool (strict)"("Disabled"=w600) -> ()  [unwired: 2 in, 2 out]
        n309 = property on="Operation" class="TabCtl (strict)"("DisabledEnum"=w600) -> ()  [unwired: 2 in, 2 out]
        n310 = property on="Save Masks" class="Bool"("DisabledEnum"=w596) -> ()  [unwired: 2 in, 2 out]
        n311 = property on="Get Masks" class="Bool (strict)"("DisabledEnum"=w596) -> ()  [unwired: 2 in, 2 out]
      }
      frame "Pre-Mask Ctrl" {
        # "0: Pre-Mask - DAQmx  \n1: Pre-Mask - Prior\n2: Pre-Mask - SW\n3: Mask Ctrl (Bool 1, T)"
        n312 = for {
          N: 5 -> [_]
          tunnel: [w616] -> w609 mode=indexing
          i -> [w617]
          n313 = case shown="0" w617 {
            tunnel: T9 {"Exec States"=enum."SW Init", "U32"=0, "I32"=0, "DBL_1 (X)"=0.0, "DBL_2 (Y)"=0.0, "DBL_3 (Z)"=0.0, "Bool_1"=FALSE, "Bool_2"=FALSE, "Variant"=variant(string "")} ("Que") -> [w621 w624 w627 w631 w634]
            tunnel: [w620 w623 w626 w630 w633] -> w616
            frame 0 {
              n314 = Bundle By Name(cluster=w621, "Exec States"=Image-DO_with_Stage_-_Exec_States."Pre-Mask HW - DAQmx") -> (w620:T9)
            }
            frame 1 {
              n315 = Bundle By Name(cluster=w624, "Exec States"=Image-DO_with_Stage_-_Exec_States."Pre-Mask HW - Prior") -> (w623:T9)
            }
            frame 2 {
              n316 = Bundle By Name(cluster=w627, "Exec States"=Image-DO_with_Stage_-_Exec_States."Pre-Mask SW") -> (w626:T9)
            }
            frame 3 {
              n317 = Bundle By Name(cluster=w631, "Exec States"=Image-DO_with_Stage_-_Exec_States."Mask Crtl", "Bool_1"=TRUE) -> (w630:T9)
            }
            frame Default {
              # "Invalid case"
              n318 = Bundle By Name(cluster=w634, "Exec States"=Image-DO_with_Stage_-_Exec_States."Wait (ms)") -> (w633:T9)
            }
          }
        }
        n319 = call "Image-DO with Stage - Que Actions.vi"("Actions"=w609, "Qqu Ref In"=w611) -> ("Que Ref Out"=w610:refnum<queue>)  [unwired: 8 in, 1 out]
      }
      frame "Pre-Mask HW - DAQmx" {
        n320 = property on="Statice DO" class="Arr (strict)"() -> ("Visible"=w638:bool, "Value"=w635:bool[])  [unwired: 2 in, 2 out]
        n321 = case shown="True" w638 {
          tunnel: w636 -> [w642 w646]
          tunnel: [w642 w645] -> w637
          tunnel: w635 -> [_ w644]
          frame False {
          }
          frame True {
            n322 = Boolean Array To Number(Boolean array=w644) -> (number=w643:u32)
            n323 = call "Image-DO with Stage - Set Static DO.vi"("Action"=T21."Write Lnes", "error in"=w646, "line data"=w643) -> ("error out"=w645:errorcluster)  [unwired: 8 in]
          }
        }
      }
      frame "Pre-Mask HW - Prior".."Pre-Mask HW - Reserved 2" {
        # "Place Holder"
      }
      frame "Pre-Mask SW" {
        w652 = u8 2 ("Disabled")
        # "Masks collected at only the first point of a z scan"
        n324 = local read "Z Scan Parameters"() -> (w668:T8)
        n325 = local read "Dwell Time (sec)"() -> (w667:dbl)
        n326 = local read "Cycle Time (sec)"() -> (w666:dbl)
        n327 = local read "Grid Parameters"() -> (w669:T7)
        n328 = local read "XY Scan Mode"() -> (w653:bool)
        n329 = Bundle By Name(cluster=T23 {"Grid"={"X Axis"={"Start Pt"=0.0, "Step Size"=100.0, "# Steps"=12}, "Y Axis"={"Start Pt"=20.0, "Step Size"=2.0, "# Steps"=2}, "Pattern"=enum."Bidirectional Raster", "Major Axis"=FALSE}, "Z Scan"={"Z Axis"={"Start Pt"=100.0, "Step Size"=20.0, "# Steps"=0}, "Pattern"=enum."Unidirectional Raster", "Active"=FALSE}, "XY Scan Mode"=FALSE, "Dwell Time"=0.0, "Cycle Time"=1.0} ("Stage Paramaters"), "Grid"=w669, "Z Scan"=w668, "Z Scan.Active"=FALSE ("XY Scan Mode"), "Dwell Time"=w667, "Cycle Time"=w666, "XY Scan Mode"=w653) -> (w661:T23)
        n330 = local read "Imageing Parameters"() -> (w659:T2)
        n331 = call "Image-DO with Stage - User Defined Pts.vi"() -> ("User Defined Pts Out"=w670:T6[])  [unwired: 8 in, 3 out]
        n332 = call "Image-DO with Stage - Stage Position.vi"("Action"=T22."Load Points", "Stage Scan Paramaters"=w661, "User Defined Pts"=w670) -> ("Position Info"=w658:T28)  [unwired: 4 in, 4 out]
        n333 = call "Image-DO with Stage - User GUI Settings.vi"("Action (0: Read All)"=T11."Set Stage Settings", "Stage Settings In"=w661) -> ()  [unwired: 8 in, 6 out]
        n334 = Unbundle By Name(w659) -> ("X Mirror.# Pixels"=w656:i32, "Y Mirror.# Pixels"=w655:i32)
        n335 = Unbundle By Name(w658) -> ("# XY Steps"=w657:i32)
        n336 = Bundle("# XY Steps"=w657, "# Pixels"=w656, "# Pixels"=w655) -> (w654:T29)  [unwired: 1 in]
        n337 = local read "Step Mode"() -> (w679:bool)
        n338 = call "Image-DO with Stage - DO Masks.vi"("Action"=T19."Init Scan Masks", "Scan Mask Size"=w654) -> ()  [unwired: 8 in, 2 out]
        n339 = local write "Status"("** Starting Mask Scan **" ("Status")) -> ()
        n340 = property on="Advance" class="Bool (strict)"("Blinking"=w679, "DisabledEnum"=0) -> ()  [unwired: 2 in, 2 out]
        n341 = property on="Get Masks" class="Bool (strict)"("Blinking"=TRUE) -> ()  [unwired: 2 in, 2 out]
        n342 = call "Image-DO with Stage - System State.vi"("Set State (F:Get)"=TRUE ("Action (F:Get)"), "Sys State In"=Image-DO_with_Stage_-_Sys_State."Masking") -> ()  [unwired: 7 in, 3 out]
        n343 = call "Image-DO with Stage - User GUI Settings.vi"("Action (0: Read All)"=T11."Set Descriptor", "File Descriptor In"="") -> ()  [unwired: 8 in, 6 out]
        n344 = property on="Exit" class="Bool"("Disabled"=w652) -> ()  [unwired: 2 in, 2 out]
        n345 = property on="Aquire Image" class="Bool (strict)"("DisabledEnum"=w652) -> ()  [unwired: 2 in, 2 out]
        n346 = property on="Get Image Mask" class="Bool"("DisabledEnum"=w652) -> ()  [unwired: 2 in, 2 out]
        n347 = property on="Save Masks" class="Bool"("DisabledEnum"=w652) -> ()  [unwired: 2 in, 2 out]
        n348 = property on="Common Mask" class="Bool (strict)"("DisabledEnum"=w652) -> ()  [unwired: 2 in, 2 out]
        n349 = property on="Scan" class="Bool (strict)"("DisabledEnum"=w652) -> ()  [unwired: 2 in, 2 out]
        n350 = property on="Save Image" class="Bool"("DisabledEnum"=w652) -> ()  [unwired: 2 in, 2 out]
        n351 = property on="Reset I/O" class="Bool"("DisabledEnum"=w652) -> ()  [unwired: 2 in, 2 out]
        n352 = property on="Auto Save" class="Bool (strict)"("Disabled"=w652) -> ()  [unwired: 2 in, 2 out]
        n353 = property on="Operation" class="TabCtl (strict)"("DisabledEnum"=w652, "Value"=enum32{"Imaging", "Stage Scan"}."Stage Scan" ("Operation")) -> ()  [unwired: 2 in, 2 out]
      }
      frame "Mask Crtl" {
        # "First Call"
        n354 = Unbundle By Name(w691) -> ("Bool_1"=w685:bool)
        n355 = case shown="True" "Get Masks" {
          tunnel: [w695 w710] -> w686
          tunnel: [T9[] [{"Exec States"=enum."Post-Mask Crtl", "U32"=0, "I32"=0, "DBL_1 (X)"=0.0, "DBL_2 (Y)"=0.0, "DBL_3 (Z)"=0.0, "Bool_1"=FALSE, "Bool_2"=FALSE, "Variant"=variant}] ("Actions") w709] -> w687
          tunnel: w685 -> [_ w699]
          tunnel: "Common Mask" -> [_ w701]
          frame False {
            # "0: Post Scan Ctrl"
            n356 = local read "Status"() -> (w695:string)
          }
          frame True {
            # "Waiting on User"
            n357 = property on="Advance" class="Bool (strict)"() -> ("Blinking"=w703:bool)  [unwired: 2 in, 2 out]
            n358 = local read "Estmated Frame Time"() -> (w707:dbl)
            n359 = local read "Step Mode"() -> (w704:bool)
            n360 = local read "Advance"() -> (w702:bool)
            n361 = Select(t=w702, s=w703, f=TRUE) -> (s? t:f=w700:bool)
            n362 = Select(t=TRUE, s=w699, f=w700) -> (s? t:f=w697:bool)
            n363 = Multiply(x=2.0, y=w707) -> (x*y=w705:dbl)
            n364 = case shown="True" w697 {
              tunnel: ["Waiting on use to select \"Advance\" scan." ("Status") w732] -> w710
              tunnel: [w713 w731] -> w709
              tunnel: w699 -> [w711 w730]
              tunnel: w704 -> [_ _]
              tunnel: w705 -> [w712 w729]
              tunnel: w701 -> [_ w727]
              frame False {
                w720 = T9 {"Exec States"=enum."Post-Scan Crtl", "U32"=0, "I32"=0, "DBL_1 (X)"=0.0, "DBL_2 (Y)"=0.0, "DBL_3 (Z)"=0.0, "Bool_1"=FALSE, "Bool_2"=FALSE, "Variant"=variant}
                # "Step Mode: On\nWaiting on User"
                n365 = Bundle By Name(cluster=w720, "Exec States"=Image-DO_with_Stage_-_Exec_States."Start Imaging - DAQmx") -> (w718:T9)
                n366 = Bundle By Name(cluster=w720, "Exec States"=Image-DO_with_Stage_-_Exec_States."Read Images - DAQmx", "DBL_1 (X)"=w712) -> (w717:T9)
                n367 = Bundle By Name(cluster=w720, "Exec States"=Image-DO_with_Stage_-_Exec_States."Stop Imaging - DAQmx") -> (w716:T9)
                n368 = Bundle By Name(cluster=w720, "Exec States"=Image-DO_with_Stage_-_Exec_States."Display Image", "Bool_1"=FALSE) -> (w715:T9)
                n369 = Bundle By Name(cluster=w720, "Exec States"=Image-DO_with_Stage_-_Exec_States."Mask Crtl", "Bool_1"=w711) -> (w714:T9)
                n370 = call <vilib>:"Beep.vi"() -> ()  [unwired: 12 in]
                n371 = Build Array(w718, w717, w716, w715, w714) -> (w713:T9[])
              }
              frame True {
                # "Advance"
                n372 = call "Image-DO with Stage - Mask Ctrl Logic.vi"("Image Timeout (-1)"=w729, "Common Mask"=w727, "First Call"=w730) -> ("Status"=w732:string, "Actions"=w731:T9[])  [unwired: 7 in]
                n373 = local write "Advance"(FALSE ("Advance")) -> ()
              }
            }
          }
        }
        n374 = local write "Status"(w686) -> ()
        n375 = call "Image-DO with Stage - Que Actions.vi"("Actions"=w687, "Qqu Ref In"=w690) -> ("Que Ref Out"=w689:refnum<queue>)  [unwired: 8 in, 1 out]
      }
      frame "Post-Mask Crtl" {
        # "0: Post-Mask - DAQmx - AO\n1: Post-Mask - Prior\n2: Post-Mask - SW"
        n376 = call "Image-DO with Stage - Que Actions.vi"("Actions"=T9[] [{"Exec States"=enum."Post-Mask HW - DAQmx", "U32"=0, "I32"=0, "DBL_1 (X)"=0.0, "DBL_2 (Y)"=0.0, "DBL_3 (Z)"=0.0, "Bool_1"=FALSE, "Bool_2"=FALSE, "Variant"=variant(string "")}, {"Exec States"=enum."Post-Mask HW - Prior", "U32"=0, "I32"=0, "DBL_1 (X)"=0.0, "DBL_2 (Y)"=0.0, "DBL_3 (Z)"=0.0, "Bool_1"=FALSE, "Bool_2"=FALSE, "Variant"=variant(string "")}, {"Exec States"=enum."Post-Mask SW", "U32"=0, "I32"=0, "DBL_1 (X)"=0.0, "DBL_2 (Y)"=0.0, "DBL_3 (Z)"=0.0, "Bool_1"=FALSE, "Bool_2"=FALSE, "Variant"=variant(string "")}], "Qqu Ref In"=w734) -> ("Que Ref Out"=w733:refnum<queue>)  [unwired: 8 in, 1 out]
      }
      frame "Post-Mask HW - DAQmx" {
        n377 = property on="Statice DO" class="Arr (strict)"() -> ("Visible"=w741:bool)  [unwired: 2 in, 2 out]
        n378 = case shown="True" w741 {
          tunnel: w740 -> [w745 w747]
          tunnel: [w745 w746] -> w739
          frame False {
          }
          frame True {
            n379 = call "Image-DO with Stage - Set Static DO.vi"("Action"=T21."Write Lnes", "error in"=w747, "line data"=u8 0) -> ("error out"=w746:errorcluster)  [unwired: 8 in]
          }
        }
      }
      frame "Post-Mask HW - Prior".."Post-Mask HW - Reserved 2" {
        # "Place Holder"
      }
      frame "Post-Mask SW" {
        w768 = FALSE ("Blinking")
        w754 = u8 0 ("Disabled")
        n380 = local read "Status"() -> (w756:string)
        n381 = call "Image-DO with Stage - System State.vi"("Set State (F:Get)"=TRUE ("Action (F:Get)"), "Sys State In"=Image-DO_with_Stage_-_Sys_State."Configured") -> ()  [unwired: 7 in, 3 out]
        n382 = call "Image-DO with Stage - User GUI Settings.vi"("Action (0: Read All)"=T11."Set Descriptor", "File Descriptor In"="") -> ()  [unwired: 8 in, 6 out]
        n383 = Search/Split String(string=w756, search string/char (-)="\nPos") -> (match + rest of string=w755:string)  [unwired: 1 in, 2 out]
        n384 = property on="Get Masks" class="Bool (strict)"() -> (error out=w769:errorcluster, "Value"=w770:bool)  [unwired: 2 in, 1 out]
        n385 = Concatenate Strings("** Mask Scan stopped at **" ("Status"), w755) -> (w759:string)
        n386 = Select(t="** Mask Scan Complete**" ("Status"), s=w770, f=w759) -> (s? t:f=w758:string)
        n387 = property on="Advance" class="Bool (strict)"("Blinking"=FALSE, "DisabledEnum"=2) -> ()  [unwired: 2 in, 2 out]
        n388 = property on="Get Masks" class="Bool (strict)"(error in=w769, "Blinking"=w768, "Value"=w768) -> ()  [unwired: 1 in, 2 out]
        n389 = local write "Status"(w758) -> ()
        n390 = property on="Exit" class="Bool"("Disabled"=w754) -> ()  [unwired: 2 in, 2 out]
        n391 = property on="Aquire Image" class="Bool (strict)"("DisabledEnum"=w754) -> ()  [unwired: 2 in, 2 out]
        n392 = property on="Save Masks" class="Bool"("DisabledEnum"=w754) -> ()  [unwired: 2 in, 2 out]
        n393 = property on="Get Image Mask" class="Bool"("DisabledEnum"=w754) -> ()  [unwired: 2 in, 2 out]
        n394 = property on="Common Mask" class="Bool (strict)"("DisabledEnum"=w754) -> ()  [unwired: 2 in, 2 out]
        n395 = property on="Scan" class="Bool (strict)"("DisabledEnum"=w754) -> ()  [unwired: 2 in, 2 out]
        n396 = property on="Save Image" class="Bool"("DisabledEnum"=w754) -> ()  [unwired: 2 in, 2 out]
        n397 = property on="Reset I/O" class="Bool"("DisabledEnum"=w754) -> ()  [unwired: 2 in, 2 out]
        n398 = property on="Auto Save" class="Bool (strict)"("Disabled"=w754) -> ()  [unwired: 2 in, 2 out]
        n399 = property on="Operation" class="TabCtl (strict)"("DisabledEnum"=w754) -> ()  [unwired: 2 in, 2 out]
      }
      frame "Pre-Scan Ctrl" {
        # "Configure Imaging - DAQmx\n  - I32: Mask Index\n  - Bool 1\n        T: Continuous Mode\n         F: Finite Mode\n\nSave File\n  - Bool1: Append Parameters\n  - Bool2: Mask Save\n        T: Image Mask\n        F: Scan Masks\n  - Variant: File Operation"
        # "0: Pre-Scan - DAQmx  \n1: Pre-Scan - Prior\n2: Pre-Scan - SW\n3: Save Parameter File  / Wait\n4: Open Data File  / Wait\n5: Scan Ctrl (Bool 1, T)"
        n400 = for {
          N: 6 -> [_]
          tunnel: [w782] -> w776 mode=indexing
          i -> [w783]
          n401 = case shown="5" w783 {
            tunnel: T9 {"Exec States"=enum."SW Init", "U32"=0, "I32"=0, "DBL_1 (X)"=0.0, "DBL_2 (Y)"=0.0, "DBL_3 (Z)"=0.0, "Bool_1"=FALSE, "Bool_2"=FALSE, "Variant"=variant(string "")} ("Que") -> [w787 w790 w793 w797 w806 w815 w818]
            tunnel: [w786 w789 w792 w796 w805 w814 w817] -> w782
            frame 0 {
              n402 = Bundle By Name(cluster=w787, "Exec States"=Image-DO_with_Stage_-_Exec_States."Pre-Scan HW - DAQmx") -> (w786:T9)
            }
            frame 1 {
              n403 = Bundle By Name(cluster=w790, "Exec States"=Image-DO_with_Stage_-_Exec_States."Pre-Scan HW - Prior") -> (w789:T9)
            }
            frame 2 {
              n404 = Bundle By Name(cluster=w793, "Exec States"=Image-DO_with_Stage_-_Exec_States."Pre-Scan SW") -> (w792:T9)
            }
            frame 3 {
              n405 = local read "Auto Save"() -> (w802:bool)
              n406 = Select(t=Image-DO_with_Stage_-_Exec_States."Save Files" ("Exec States"), s=w802, f=Image-DO_with_Stage_-_Exec_States."Wait (ms)" ("Exec States")) -> (s? t:f=w801:T10)
              n407 = To Variant(anything=Image-DO_with_Stage_-_File_Save_Option."Save Scan Parameters" ("Action")) -> (Variant=w800:variant)
              n408 = Bundle By Name(cluster=w797, "Exec States"=w801, "Variant"=w800, "Bool_1"=FALSE) -> (w796:T9)
            }
            frame 4 {
              n409 = local read "Auto Save"() -> (w811:bool)
              n410 = Select(t=Image-DO_with_Stage_-_Exec_States."Save Files" ("Exec States"), s=w811, f=Image-DO_with_Stage_-_Exec_States."Wait (ms)" ("Exec States")) -> (s? t:f=w810:T10)
              n411 = To Variant(anything=Image-DO_with_Stage_-_File_Save_Option."Open Data Files" ("Action")) -> (Variant=w809:variant)
              n412 = Bundle By Name(cluster=w806, "Exec States"=w810, "Variant"=w809, "Bool_1"=FALSE) -> (w805:T9)
            }
            frame 5 {
              n413 = Bundle By Name(cluster=w815, "Exec States"=Image-DO_with_Stage_-_Exec_States."Scan Ctrl", "Bool_1"=TRUE) -> (w814:T9)
            }
            frame Default {
              # "Invalid case"
              n414 = Bundle By Name(cluster=w818, "Exec States"=Image-DO_with_Stage_-_Exec_States."Wait (ms)") -> (w817:T9)
            }
          }
        }
        n415 = call "Image-DO with Stage - Que Actions.vi"("Actions"=w776, "Qqu Ref In"=w779) -> ("Que Ref Out"=w778:refnum<queue>)  [unwired: 8 in, 1 out]
      }
      frame "Pre-Scan HW - DAQmx" {
        n416 = property on="Statice DO" class="Arr (strict)"() -> ("Visible"=w822:bool, "Value"=w819:bool[])  [unwired: 2 in, 2 out]
        n417 = case shown="True" w822 {
          tunnel: w821 -> [w826 w830]
          tunnel: [w826 w829] -> w820
          tunnel: w819 -> [_ w828]
          frame False {
          }
          frame True {
            n418 = Boolean Array To Number(Boolean array=w828) -> (number=w827:u32)
            n419 = call "Image-DO with Stage - Set Static DO.vi"("Action"=T21."Write Lnes", "error in"=w830, "line data"=w827) -> ("error out"=w829:errorcluster)  [unwired: 8 in]
          }
        }
      }
      frame "Pre-Scan HW - Prior".."Pre-Scan HW - Reserve 2" {
        # "Place Holder"
      }
      frame "Pre-Scan SW" {
        w838 = u8 2 ("Disabled")
        # "Pre-configure the data space and GUI for data acquisition."
        n420 = Bundle By Name(cluster=T23 {"Grid"={"X Axis"={"Start Pt"=0.0, "Step Size"=100.0, "# Steps"=12}, "Y Axis"={"Start Pt"=20.0, "Step Size"=2.0, "# Steps"=2}, "Pattern"=enum."Bidirectional Raster", "Major Axis"=FALSE}, "Z Scan"={"Z Axis"={"Start Pt"=100.0, "Step Size"=20.0, "# Steps"=0}, "Pattern"=enum."Unidirectional Raster", "Active"=FALSE}, "XY Scan Mode"=FALSE, "Dwell Time"=0.0, "Cycle Time"=1.0} ("Stage Paramaters"), "Grid"="Grid Parameters", "Z Scan"="Z Scan Parameters", "XY Scan Mode"="XY Scan Mode", "Dwell Time"="Dwell Time (sec)", "Cycle Time"="Cycle Time (sec)") -> (w842:T23)
        n421 = call "Image-DO with Stage - User GUI Settings.vi"("Action (0: Read All)"=T11."Set Descriptor", "File Descriptor In"="") -> ()  [unwired: 8 in, 6 out]
        n422 = call "Image-DO with Stage - System State.vi"("Set State (F:Get)"=TRUE ("Action (F:Get)"), "Sys State In"=Image-DO_with_Stage_-_Sys_State."Scanning") -> ()  [unwired: 7 in, 3 out]
        n423 = call "Image-DO with Stage - User Defined Pts.vi"() -> ("User Defined Pts Out"=w848:T6[])  [unwired: 8 in, 3 out]
        n424 = local read "Common Mask"() -> (w836:bool)
        n425 = call "Image-DO with Stage - Stage Position.vi"("Action"=T22."Load Points", "Stage Scan Paramaters"=w842, "User Defined Pts"=w848) -> ("Position Info"=w837:T28)  [unwired: 4 in, 4 out]
        n426 = call "Image-DO with Stage - User GUI Settings.vi"("Action (0: Read All)"=T11."Set Stage Settings", "Stage Settings In"=w842) -> ()  [unwired: 8 in, 6 out]
        n427 = local read "Step Mode"() -> (w853:bool)
        n428 = case shown="True" w836 {
          tunnel: w837 -> [_ w864]
          frame False {
          }
          frame True {
            n429 = Unbundle By Name(w864) -> ("# XY Steps"=w862:i32)
            n430 = call "Image-DO with Stage - DO Masks.vi"() -> ("Image Mask Out"=w863:u8[][])  [unwired: 10 in, 1 out]
            n431 = call "Image-DO with Stage - DO Masks.vi"("Action"=T19."Init Scan Masks", "Scan Mask Index"=w862, "Image Mask"=w863) -> ()  [unwired: 7 in, 2 out]
          }
        }
        n432 = property on="Advance" class="Bool (strict)"("Blinking"=w853, "DisabledEnum"=0) -> ()  [unwired: 2 in, 2 out]
        n433 = local write "Status"("Starting Scan" ("Status")) -> ()
        n434 = property on="Scan" class="Bool (strict)"("Blinking"=TRUE) -> ()  [unwired: 2 in, 2 out]
        n435 = property on="Exit" class="Bool"("Disabled"=w838) -> ()  [unwired: 2 in, 2 out]
        n436 = property on="Aquire Image" class="Bool (strict)"("DisabledEnum"=w838) -> ()  [unwired: 2 in, 2 out]
        n437 = property on="Get Image Mask" class="Bool"("DisabledEnum"=w838) -> ()  [unwired: 2 in, 2 out]
        n438 = property on="Get Masks" class="Bool (strict)"("DisabledEnum"=w838) -> ()  [unwired: 2 in, 2 out]
        n439 = property on="Save Masks" class="Bool"("DisabledEnum"=w838) -> ()  [unwired: 2 in, 2 out]
        n440 = property on="Common Mask" class="Bool (strict)"("DisabledEnum"=w838) -> ()  [unwired: 2 in, 2 out]
        n441 = property on="Save Image" class="Bool"("DisabledEnum"=w838) -> ()  [unwired: 2 in, 2 out]
        n442 = property on="Reset I/O" class="Bool"("DisabledEnum"=w838) -> ()  [unwired: 2 in, 2 out]
        n443 = property on="Auto Save" class="Bool (strict)"("Disabled"=w838) -> ()  [unwired: 2 in, 2 out]
        n444 = property on="Operation" class="TabCtl (strict)"("DisabledEnum"=w838, "Value"=enum32{"Imaging", "Stage Scan"}."Stage Scan" ("Operation")) -> ()  [unwired: 2 in, 2 out]
      }
      frame "Scan Ctrl" {
        # "First Call"
        n445 = Unbundle By Name(w871) -> ("Bool_1"=w870:bool)
        n446 = case shown="True" "Scan" {
          tunnel: w870 -> [_ w882]
          tunnel: "Auto Save" -> [_ w891]
          tunnel: [w877 w890] -> w868
          tunnel: [T9[] [{"Exec States"=enum."Post-Scan Crtl", "U32"=0, "I32"=0, "DBL_1 (X)"=0.0, "DBL_2 (Y)"=0.0, "DBL_3 (Z)"=0.0, "Bool_1"=FALSE, "Bool_2"=FALSE, "Variant"=variant}] ("Actions") w889] -> w867
          frame False {
            # "0: Post Scan Ctrl"
            n447 = local read "Status"() -> (w877:string)
          }
          frame True {
            # "Waiting on User"
            n448 = local read "Estmated Frame Time"() -> (w886:dbl)
            n449 = Select(t="Advance", s="Step Mode", f=TRUE) -> (s? t:f=w883:bool)
            n450 = Multiply(x=2.0, y=w886) -> (x*y=w884:dbl)
            n451 = Select(t=TRUE, s=w882, f=w883) -> (s? t:f=w881:bool)
            n452 = case shown="True" w881 {
              tunnel: w891 -> [_ w913]
              tunnel: ["Waiting on use to select \"Advance\" scan." ("Status") w912] -> w890
              tunnel: [w893 w911] -> w889
              tunnel: w882 -> [w899 w910]
              tunnel: w884 -> [w892 w909]
              frame False {
                w901 = T9 {"Exec States"=enum."Post-Scan Crtl", "U32"=0, "I32"=0, "DBL_1 (X)"=0.0, "DBL_2 (Y)"=0.0, "DBL_3 (Z)"=0.0, "Bool_1"=FALSE, "Bool_2"=FALSE, "Variant"=variant}
                # "Step Mode: On\nWaiting on User"
                n453 = Bundle By Name(cluster=w901, "Exec States"=Image-DO_with_Stage_-_Exec_States."Start Imaging - DAQmx") -> (w898:T9)
                n454 = Bundle By Name(cluster=w901, "Exec States"=Image-DO_with_Stage_-_Exec_States."Read Images - DAQmx", "DBL_1 (X)"=w892) -> (w897:T9)
                n455 = Bundle By Name(cluster=w901, "Exec States"=Image-DO_with_Stage_-_Exec_States."Stop Imaging - DAQmx") -> (w896:T9)
                n456 = Bundle By Name(cluster=w901, "Exec States"=Image-DO_with_Stage_-_Exec_States."Display Image", "Bool_1"=FALSE) -> (w895:T9)
                n457 = Bundle By Name(cluster=w901, "Exec States"=Image-DO_with_Stage_-_Exec_States."Scan Ctrl", "Bool_1"=w899) -> (w894:T9)
                n458 = call <vilib>:"Beep.vi"() -> ()  [unwired: 12 in]
                n459 = Build Array(w898, w897, w896, w895, w894) -> (w893:T9[])
              }
              frame True {
                # "Advance"
                n460 = call "Image-DO with Stage - Scan Ctrl Logic.vi"("Image Timeout (-1)"=w909, "Auto Save"=w913, "First Call"=w910) -> ("Status"=w912:string, "Actions"=w911:T9[])  [unwired: 7 in]
                n461 = local write "Advance"(FALSE ("Advance")) -> ()
              }
            }
          }
        }
        "Status" <- w868
        n462 = call "Image-DO with Stage - Que Actions.vi"("Actions"=w867, "Qqu Ref In"=w873) -> ("Que Ref Out"=w874:refnum<queue>)  [unwired: 8 in, 1 out]
      }
      frame "Post-Scan Crtl" {
        # "Save File\n  - Bool1: Append Parameters\n  - Bool2: Mask Save\n        T: Image Mask\n        F: Scan Masks\n  - Variant: File Operation"
        # "0: Post-Scan - DAQmx  \n1: Post-Scan - Prior\n2: Post-Scan - SW\n3: Close Data File  / Wait (BL1: T)"
        n463 = for {
          N: 4 -> [_]
          tunnel: [w921] -> w914 mode=indexing
          i -> [w922]
          n464 = case shown="3" w922 {
            tunnel: T9 {"Exec States"=enum."SW Init", "U32"=0, "I32"=0, "DBL_1 (X)"=0.0, "DBL_2 (Y)"=0.0, "DBL_3 (Z)"=0.0, "Bool_1"=FALSE, "Bool_2"=FALSE, "Variant"=variant(string "")} ("Que") -> [w926 w929 w932 w937 w945]
            tunnel: [w925 w928 w931 w936 w944] -> w921
            frame 0 {
              n465 = Bundle By Name(cluster=w926, "Exec States"=Image-DO_with_Stage_-_Exec_States."Post-Scan HW - DAQmx") -> (w925:T9)
            }
            frame 1 {
              n466 = Bundle By Name(cluster=w929, "Exec States"=Image-DO_with_Stage_-_Exec_States."Post-Scan HW - Prior") -> (w928:T9)
            }
            frame 2 {
              n467 = Bundle By Name(cluster=w932, "Exec States"=Image-DO_with_Stage_-_Exec_States."Post-Scan SW") -> (w931:T9)
            }
            frame 3 {
              n468 = local read "Auto Save"() -> (w942:bool)
              n469 = Select(t=Image-DO_with_Stage_-_Exec_States."Save Files" ("Exec States"), s=w942, f=Image-DO_with_Stage_-_Exec_States."Wait (ms)" ("Exec States")) -> (s? t:f=w941:T10)
              n470 = To Variant(anything=Image-DO_with_Stage_-_File_Save_Option."Close Data Files" ("Action")) -> (Variant=w940:variant)
              n471 = Bundle By Name(cluster=w937, "Exec States"=w941, "Variant"=w940, "Bool_1"=TRUE, "Bool_2"=FALSE) -> (w936:T9)
            }
            frame Default {
              # "Invalid case"
              n472 = Bundle By Name(cluster=w945, "Exec States"=Image-DO_with_Stage_-_Exec_States."Wait (ms)") -> (w944:T9)
            }
          }
        }
        n473 = call "Image-DO with Stage - Que Actions.vi"("Actions"=w914, "Qqu Ref In"=w918) -> ("Que Ref Out"=w917:refnum<queue>)  [unwired: 8 in, 1 out]
      }
      frame "Post-Scan HW - DAQmx" {
        n474 = property on="Statice DO" class="Arr (strict)"() -> ("Visible"=w948:bool)  [unwired: 2 in, 2 out]
        n475 = case shown="True" w948 {
          tunnel: w946 -> [w952 w954]
          tunnel: [w952 w953] -> w947
          frame False {
          }
          frame True {
            n476 = call "Image-DO with Stage - Set Static DO.vi"("Action"=T21."Write Lnes", "error in"=w954, "line data"=u8 0) -> ("error out"=w953:errorcluster)  [unwired: 8 in]
          }
        }
      }
      frame "Post-Scan HW - Prior".."Post-Scan HW - Reserve 2" {
        # "Place Holder"
      }
      frame "Post-Scan SW" {
        w973 = FALSE ("Blinking")
        w961 = u8 0 ("Disabled")
        n477 = call "Image-DO with Stage - System State.vi"("Set State (F:Get)"=TRUE ("Action (F:Get)"), "Sys State In"=Image-DO_with_Stage_-_Sys_State."Configured") -> ()  [unwired: 7 in, 3 out]
        n478 = call "Image-DO with Stage - User GUI Settings.vi"("Action (0: Read All)"=T11."Set Descriptor", "File Descriptor In"="") -> ()  [unwired: 8 in, 6 out]
        n479 = local read "Status"() -> (w967:string)
        n480 = Search/Split String(string=w967, search string/char (-)="\nPos") -> (match + rest of string=w966:string)  [unwired: 1 in, 2 out]
        n481 = property on="Scan" class="Bool (strict)"() -> (error out=w972:errorcluster, "Value"=w977:bool)  [unwired: 2 in, 1 out]
        n482 = Concatenate Strings("** Scanning stopped at **" ("Status"), w966) -> (w970:string)
        n483 = Select(t="** Scanning Complete **" ("Status"), s=w977, f=w970) -> (s? t:f=w969:string)
        n484 = property on="Advance" class="Bool (strict)"("Blinking"=FALSE, "DisabledEnum"=2) -> ()  [unwired: 2 in, 2 out]
        n485 = property on="Scan" class="Bool (strict)"(error in=w972, "Blinking"=w973, "Value"=w973) -> ()  [unwired: 1 in, 2 out]
        n486 = local write "Status"(w969) -> ()
        n487 = local read "Common Mask"() -> (w964:bool)
        n488 = Select(t=u8 2 ("Disabled"), s=w964, f=u8 0) -> (s? t:f=w965:u8)
        n489 = property on="Exit" class="Bool"("Disabled"=w961) -> ()  [unwired: 2 in, 2 out]
        n490 = property on="Aquire Image" class="Bool (strict)"("DisabledEnum"=w961) -> ()  [unwired: 2 in, 2 out]
        n491 = property on="Get Image Mask" class="Bool"("DisabledEnum"=w961) -> ()  [unwired: 2 in, 2 out]
        n492 = property on="Save Image" class="Bool"("DisabledEnum"=w961) -> ()  [unwired: 2 in, 2 out]
        n493 = property on="Reset I/O" class="Bool"("DisabledEnum"=w961) -> ()  [unwired: 2 in, 2 out]
        n494 = property on="Auto Save" class="Bool (strict)"("Disabled"=w961) -> ()  [unwired: 2 in, 2 out]
        n495 = property on="Operation" class="TabCtl (strict)"("DisabledEnum"=w961) -> ()  [unwired: 2 in, 2 out]
        n496 = property on="Common Mask" class="Bool (strict)"("DisabledEnum"=w961) -> ()  [unwired: 2 in, 2 out]
        n497 = property on="Save Masks" class="Bool"("DisabledEnum"=w965) -> ()  [unwired: 2 in, 2 out]
        n498 = property on="Get Masks" class="Bool (strict)"("DisabledEnum"=w965) -> ()  [unwired: 2 in, 2 out]
      }
      frame "Wait (ms)" {
        n499 = Unbundle By Name(w989) -> ("U32"=w988:u32)
        n500 = Wait (ms)(milliseconds to wait=w988) -> ()  [unwired: 1 out]
      }
      frame "Confgure Imaging - DAQmx" {
        w1005 = TRUE ("Action (F:Get)")
        w1007 = Imager_-_Scan_Starting_Point."X-Min, Y-Min" ("Starting Pt")
        w1017 = 10123 items=["Finite Samples"=10178, "Continuous Samples"=10123, "Hardware Timed Single Point"=12522] ("Sample Mode")
        w1018 = 10178 items=["Finite Samples"=10178, "Continuous Samples"=10123, "Hardware Timed Single Point"=12522] ("Sample Mode")
        # "I32: Mask Index\n\nBool 1\n   T: Continuous Mode\n    F: Finite Mode"
        n501 = Unbundle By Name(w1016) -> ("I32"=w995:i32, "Bool_1"=w1015:bool)
        n502 = Less Than 0?(x=w995) -> (x < 0?=w996:bool)
        n503 = Unbundle By Name("Imageing Parameters") -> ("Averaged"=w1012:bool, "Sample Rate"=w1011:dbl, "Pattern"=w1010:T3, "X Mirror"=w1009:T4, "Y Mirror"=w1008:T4, "Active DO lines"=w1001:T30)
        n504 = Select(t=w1017, s=w1015, f=w1018) -> (s? t:f=w1004:i32)
        n505 = Select(t=T19."Get All Mask" ("Action"), s=w996, f=T19."Get Scan Mask (n)" ("Action")) -> (s? t:f=w994:T19)
        n506 = call "Image-DO with Stage - DO Masks.vi"("Action"=w994, "Scan Mask Index"=w995) -> ("Image Mask Out"=w997:u8[][])  [unwired: 8 in, 1 out]
        n507 = Bundle By Name(cluster=T24 {"Sample Rate"=1000000.0, "Pattern"=enum."Unidirectional Raster", "Starting Pt"=enum."X-Min, Y-Max", "X Mirror"={"# Pixels"=400, "Center"=0.0, "Span"=0.1, "# Points / Pixel"=10, "Pre-Line pts"=10, "Post-Line pts"=10}, "Y Mirror"={"# Pixels"=400, "Center"=0.0, "Span"=0.1, "# Points / Pixel"=1, "Pre-Line pts"=10, "Post-Line pts"=0}} ("AO Scan Parameters"), "Starting Pt"=w1007, "Sample Rate"=w1011, "Pattern"=w1010, "X Mirror"=w1009, "Y Mirror"=w1008) -> (w1003:T24)
        n508 = Bundle By Name(cluster=T25 {"DO Port Map"={"Pixel Pattern Bit (0)"=0, "Change Pixel Bit (1)"=1, "New Line Bit (2)"=2, "In Image Bit (3)"=3, "Image Pattern Bits (4-7)"=4}, "Active DO lines"={"Pixel Pattern Bit (0)"=FALSE, "Change Pixel Bit (1)"=FALSE, "New Line Bit (2)"=FALSE, "In Image Bit (3)"=FALSE, "Image Pattern Bits (4-7)"=FALSE}, "Pixel Mask"=[], "Image Mask"=[]} ("DO Parameters"), "Active DO lines"=w1001, "Image Mask"=w997) -> (w1002:T25)
        n509 = call "Image-DO with Stage - User GUI Settings.vi"() -> ("Imaging Settings Out"=w999:T16)  [unwired: 10 in, 5 out]
        n510 = Bundle By Name(cluster=w999, "Averaged Data"=w1012, "Sample Rate"=w1011, "Pattern"=w1010, "X Mirror"=w1009, "Y Mirror"=w1008, "Starting Pt"=w1007) -> (w998:T16)
        n511 = call "Image-DO with Stage - System State.vi"("Set Mode (F:Get)"=w1005, "Set State (F:Get)"=w1005, "Sample Mode In"=w1004, "Sys State In"=Image-DO_with_Stage_-_Sys_State."Configured") -> ()  [unwired: 5 in, 3 out]
        n512 = call "Imager - Configure Image Scan.vi"("error in (no error)"=w1021, "DO Parameters"=w1002, "AO Scan Parameters"=w1003, "Sample Mode"=w1004) -> ("error out"=w1020:errorcluster)  [unwired: 5 in, 2 out]
        n513 = call "Image-DO with Stage - User GUI Settings.vi"("Action (0: Read All)"=T11."Set Image Settings", "Imaging Settings In"=w998) -> ()  [unwired: 8 in, 6 out]
      }
      frame "Start Imaging - DAQmx" {
        n514 = call "Imager - Start Imag Scan.vi"("error in (no error)"=w1026) -> ("error out"=w1025:errorcluster)  [unwired: 10 in]
      }
      frame "Read Images - DAQmx" {
        # "Timeout"
        n515 = Unbundle By Name(w1036) -> ("DBL_1 (X)"=w1032:dbl)
        n516 = call "Image-DO with Stage - User GUI Settings.vi"() -> ("Imaging Settings Out"=w1030:T16)  [unwired: 10 in, 5 out]
        n517 = Unbundle By Name(w1030) -> ("Averaged Data"=w1031:bool)
        n518 = call "Imager - Read Images.vi"("error in (no error)"=w1034, "Return Aerage (F)"=w1031, "Timeout (10 sec)"=w1032) -> ("error out"=w1035:errorcluster, "Images"=w1033:dbl[][][])  [unwired: 7 in]
      }
      frame "Wait on Image Complete - DAQmx" {
        # "Timeout"
        n519 = Unbundle By Name(w1042) -> ("DBL_1 (X)"=w1039:dbl)
        n520 = call "Imager - Wait on Image Complete.vi"("error in (no error)"=w1040, "Timeout (10 sec)"=w1039) -> ("error out"=w1041:errorcluster)  [unwired: 9 in]
      }
      frame "Stop Imaging - DAQmx" {
        n521 = call "Imager - Stop Image Scan.vi"("error in (no error)"=w1047) -> ("error out"=w1046:errorcluster)  [unwired: 10 in]
      }
      frame "Set Position - Prior" {
        n522 = case shown="True" w1057 {
          tunnel: w1055 -> [w1069 _]
          tunnel: w1059 -> [w1065 w1080]
          tunnel: [w1064 w1080] -> w1058
          frame False {
            # "Move Relative"
            n523 = Unbundle By Name(w1069) -> ("Bool_1"=w1063:bool, "DBL_1 (X)"=w1068:dbl, "DBL_2 (Y)"=w1067:dbl, "DBL_3 (Z)"=w1066:dbl)
            n524 = case shown="True" w1063 {
              tunnel: w1068 -> [w1074 w1075]
              tunnel: w1067 -> [w1073 w1076]
              tunnel: w1066 -> [w1072 w1077]
              tunnel: w1065 -> [w1071 w1079]
              tunnel: [w1070 w1078] -> w1064
              frame False {
                n525 = call "IScan Move XYZ Absolute.vi"("error in (no error)"=w1071, "Z Position"=w1072, "Y Position"=w1073, "X Position"=w1074) -> ("error out"=w1070:errorcluster)  [unwired: 2 in, 1 out]
              }
              frame True {
                n526 = call "IScan Move XYZ Relative.vi"("error in (no error)"=w1079, "Z Position"=w1077, "Y Position"=w1076, "X Position"=w1075) -> ("error out"=w1078:errorcluster)  [unwired: 2 in, 1 out]
              }
            }
          }
          frame True {
          }
        }
        n527 = Unbundle By Name(w1055) -> ("DBL_1 (X)"=w1054:dbl, "DBL_2 (Y)"=w1053:dbl, "DBL_3 (Z)"=w1052:dbl)
        n528 = Bundle By Name(cluster=T26 {"X Axis"=0.0, "Y Axis"=0.0, "Z Axis"=0.0} ("Position"), "X Axis"=w1054, "Y Axis"=w1053, "Z Axis"=w1052) -> (→"Current Position":T26)
      }
      frame "Get Position - Prior" {
        # "Update Paramater Input"
        n529 = case shown="False" w1086 {
          tunnel: w1090 -> [w1099 w1103]
          tunnel: [w1097 w1103] -> w1089
          tunnel: [w1096 w1100] -> w1084
          tunnel: [w1095 w1100] -> w1083
          tunnel: [w1094 w1100] -> w1082
          frame False {
            n530 = call "IStage Get Position.vi"("error in (no error)"=w1099) -> ("error out"=w1098:errorcluster, "YPos"=w1095:dbl, "XPos"=w1096:dbl)  [unwired: 5 in, 1 out]
            n531 = call "IZ Get Position.vi"("error in (no error)"=w1098) -> ("Position"=w1094:dbl, "error out"=w1097:errorcluster)  [unwired: 2 in]
          }
          frame True {
            n532 = call-poly <vilib>:"Random Number (Range).vi"("lower bound (0)"=u64 500, "upper bound (100)"=u64 4900) -> ("number"=w1100:dbl)  [unwired: 9 in]
          }
        }
        n533 = Unbundle By Name(w1088) -> ("Bool_1"=w1087:bool)
        n534 = Bundle By Name(cluster=T26 {"X Axis"=0.0, "Y Axis"=0.0, "Z Axis"=0.0} ("Position"), "X Axis"=w1084, "Y Axis"=w1083, "Z Axis"=w1082) -> (w1081:T26)
        n535 = case shown="True" w1087 {
          tunnel: w1084 -> [_ w1106]
          tunnel: w1083 -> [_ w1105]
          tunnel: w1082 -> [_ w1104]
          frame False {
          }
          frame True {
            n536 = local read "Z Scan Parameters"() -> (w1108:T8)
            n537 = local read "Grid Parameters"() -> (w1107:T7)
            n538 = Bundle By Name(cluster=w1108, "Z Axis.Start Pt"=w1104) -> (w1110:T8)
            n539 = Bundle By Name(cluster=w1107, "X Axis.Start Pt"=w1106, "Y Axis.Start Pt"=w1105) -> (w1109:T7)
            n540 = local write "Grid Parameters"(w1109) -> ()
            n541 = local write "Z Scan Parameters"(w1110) -> ()
          }
        }
        n542 = local write "Current Position"(w1081) -> ()
      }
      frame "Wait on Move Complete - Prior" {
        # "Timeout"
        n543 = Unbundle By Name(w1115) -> ("DBL_1 (X)"=w1114:dbl)
        n544 = case shown="False" w1111 {
          tunnel: [w1121 w1139] -> w1112
          tunnel: w1113 -> [w1120 w1139]
          tunnel: w1114 -> [w1119 _]
          frame False {
            n545 = while {
              shift-right: [w1135] -> w1121
              shift-left: w1120 -> [w1138]
              tunnel: w1119 -> [w1124]
              i -> [w1123]
              stop <- w1131 stop-if-true
              n546 = Equal To 0?(x=w1123) -> (x = 0?=w1122:bool)
              n547 = call "Elapsed Time3"("Time Target (s)"=w1124, "Reset"=w1122, "error in (no error)"=w1138) -> ("Time has Elapsed"=w1137:bool, "error out"=w1127:errorcluster)  [unwired: 9 in, 6 out]
              n548 = call "IScan Is Moving.vi"("error in (no error)"=w1127) -> ("A Moving"=w1130:bool, "Y Moving"=w1128:bool, "Z Moving"=w1129:bool, "error out"=w1126:errorcluster)  [unwired: 7 in, 4 out]
              n549 = Compound Arithmetic op=OR(w1130, w1128, w1129) -> (invert w1125:bool)
              n550 = Select(t=errorcluster {"status"=TRUE, "code"=123, "source"="Zaber Move Timeout"} ("error out"), s=w1137, f=w1126) -> (s? t:f=w1135:errorcluster)
              n551 = Compound Arithmetic op=OR(w1137, w1125, w1135) -> (w1131:bool)
              n552 = Select(t=u32 0, s=w1131, f=u32 100 ("milliseconds to wait")) -> (s? t:f=w1134:u32)
              n553 = Wait (ms)(milliseconds to wait=w1134) -> ()  [unwired: 1 out]
            }
          }
          frame True {
          }
        }
      }
      frame "Process Data" {
        # "Place Holder"
      }
      frame "Display Image" {
        # "Future Use\nData Structure\nTotal Step #\nScan Y Data\nScan X Data"
        n554 = property on="Images" class="Arr (strict)"("Val(Sgnl)"=w1144) -> ()  [unwired: 2 in, 2 out]
      }
      frame "Display Scan" {
        # "Place Holder"
      }
      frame "Save Files" {
        # "Save File\n  - Bool1: Append Parameters\n  - Bool2: Mask Save\n        T: Image Mask\n        F: Scan Masks\n  - Variant: File Operation"
        n555 = Unbundle By Name(w1175) -> ("Bool_2"=w1157:bool, "Variant"=w1172:variant, "Bool_1"=w1159:bool)
        n556 = Variant To Data(type=Image-DO_with_Stage_-_File_Save_Option."Save Image Parameters" ("Action"), Variant=w1172) -> (data=w1163:T15)  [unwired: 1 in, 1 out]
        n557 = call "Image-DO with Stage - DO Masks.vi"() -> ("Scan Masks out"=w1155:u8[][][], "Image Mask Out"=w1156:u8[][])  [unwired: 10 in]
        n558 = Build Array(w1156) -> (w1154:u8[][][])
        n559 = call "Image-DO with Stage - User GUI Settings.vi"() -> ("Path Out"=w1167:path, "Base Filename Out"=w1169:string, "File Descriptor Out"=w1168:string, "Imaging Settings Out"=w1165:T16, "# XY Positions Out"=w1164:i32, "Stage Settings Out"=w1170:T23)  [unwired: 10 in]
        n560 = Select(t=w1154, s=w1157, f=w1155) -> (s? t:f=w1153:u8[][][])
        n561 = Concatenate Strings(w1169, w1168) -> (w1166:string)
        n562 = Select(t=T27."Current File", s=w1159, f=T27."Do not append" ("Append Image Count")) -> (s? t:f=w1158:T27)
        n563 = call "Image-DO with Stage - Save Files.vi"("Path"=w1167, "Action"=w1163, "Image Mask"=w1153, "Images"=w1162, "Base Filename"=w1166, "Imaging Settings"=w1165, "Stage Settings"=w1170, "error in"=w1174, "# User Defined Positions"=w1164, "Append Image Count"=w1158, "Mask File (F:Combined)"=TRUE) -> ("error out"=w1173:errorcluster)  [unwired: 4 in]
      }
      frame "Wait on User" {
        # "Warning - Calling this case stops ALL hardware calls until the user responds or sub VI times out"
        n564 = Unbundle By Name(w1180) -> ("DBL_1 (X)"=w1188:dbl, "Bool_1"=w1189:bool)
        n565 = Greater Or Equal To 0?(x=w1188) -> (x >= 0?=w1185:bool)
        n566 = Format Into String(format string="Waiting Dwell Time \n%.0f seconds ", w1188) -> (resulting string=w1187:string)  [unwired: 2 in, 1 out]
        n567 = Select(t=w1187, s=w1185, f="Waiting on user to\npress \"Continue\".") -> (s? t:f=w1182:string)
        n568 = Select(t="Skip", s=w1185, f="Continue") -> (s? t:f=w1181:string)
        n569 = call "Wait on User.vi"("Silent (F)"=w1189, "error in (no error)"=w1179, "Timeout (Sec)"=w1188, "Boolean Text \"Continue\""=w1181, "Message String"=w1182) -> ("error out"=w1178:errorcluster)  [unwired: 4 in, 2 out]
      }
      frame "Update Mask" {
        # "I32: Mask #\nBool 1 : Common Mask"
        n570 = Unbundle By Name(w1214) -> ("Bool_1"=w1205:bool, "I32"=w1200:i32)
        n571 = Less Than 0?(x=w1200) -> (x < 0?=w1207:bool)
        n572 = Select(t=T19."Get All Mask" ("Action"), s=w1207, f=T19."Get Scan Mask (n)" ("Action")) -> (s? t:f=w1194:T19)
        n573 = call "Image-DO with Stage - User GUI Settings.vi"() -> ("Imaging Settings Out"=w1210:T16)  [unwired: 10 in, 5 out]
        n574 = call "Image-DO with Stage - DO Masks.vi"("Action"=w1194, "Scan Mask Index"=w1200) -> ("Image Mask Out"=w1206:u8[][])  [unwired: 8 in, 1 out]
        n575 = Unbundle By Name(w1210) -> ("Channel Names"=w1209:string[])
        n576 = local read "Images"() -> (w1211:dbl[][][])
        n577 = Less Than 0?(x=w1200) -> (x < 0?=w1208:bool)
        n578 = call "Digital Mask GUI - Main v1.vi"("Image Names"=w1209, "error in (no error)"=w1213, "Mask In"=w1206, "Images In"=w1211) -> ("error out"=w1212:errorcluster, "Cancelled"=w1202:bool, "Mask Out"=w1201:u8[][])  [unwired: 4 in, 1 out]
        n579 = Select(t=T19."Set Imaging Mask" ("Action"), s=w1208, f=T19."Set Scan Mask (n)" ("Action")) -> (s? t:f=w1204:T19)
        n580 = Select(t=T19."Init Scan Masks" ("Action"), s=w1205, f=w1204) -> (s? t:f=w1203:T19)
        n581 = case shown="False" w1202 {
          tunnel: w1203 -> [w1218 _]
          tunnel: w1201 -> [w1220 _]
          tunnel: w1200 -> [w1219 _]
          frame False {
            n582 = call "Image-DO with Stage - DO Masks.vi"("Action"=w1218, "Scan Mask Index"=w1219, "Image Mask"=w1220) -> ()  [unwired: 7 in, 2 out]
          }
          frame True {
            # "Canceled"
          }
        }
      }
      frame "Reserved 3".."Reserved 5" {
        # "Place Holder"
      }
      frame "HW Close Crtl" {
        # "0: HW Close - DAQmx AO\n1: HW Close - Prior\n2: HW Close - SW"
        n583 = call "Image-DO with Stage - Que Actions.vi"("Actions"=T9[] [{"Exec States"=enum."HW Close - DAQmx", "U32"=0, "I32"=0, "DBL_1 (X)"=0.0, "DBL_2 (Y)"=0.0, "DBL_3 (Z)"=0.0, "Bool_1"=FALSE, "Bool_2"=FALSE, "Variant"=variant(string "")}, {"Exec States"=enum."HW Close - Prior", "U32"=0, "I32"=0, "DBL_1 (X)"=0.0, "DBL_2 (Y)"=0.0, "DBL_3 (Z)"=0.0, "Bool_1"=FALSE, "Bool_2"=FALSE, "Variant"=variant(string "")}, {"Exec States"=enum."HW Close - SW", "U32"=0, "I32"=0, "DBL_1 (X)"=0.0, "DBL_2 (Y)"=0.0, "DBL_3 (Z)"=0.0, "Bool_1"=FALSE, "Bool_2"=FALSE, "Variant"=variant(string "")}], "Qqu Ref In"=w1228) -> ("Que Ref Out"=w1227:refnum<queue>)  [unwired: 8 in, 1 out]
      }
      frame "HW Close - DAQmx" {
        n584 = call "Imager - Clear DAQmx Tasks.vi"("error in (no error)"=w1234) -> ("error out"=w1232:errorcluster)  [unwired: 10 in]
        n585 = call "Image-DO with Stage - Set Static DO.vi"("Action"=T21."Clear Task", "error in"=w1232) -> ("error out"=w1231:errorcluster)  [unwired: 9 in]
      }
      frame "HW Close - Prior" {
        n586 = case shown="False" w1238 {
          tunnel: w1240 -> [w1245 w1248]
          tunnel: [w1244 w1248] -> w1239
          frame False {
            n587 = call "IZ Close.vi"("error in (no error)"=w1245) -> ("error out"=w1247:errorcluster)
            n588 = call "IStage Close.vi"("error in (no error)"=w1247) -> ("error out"=w1246:errorcluster)
            n589 = call "IScan Close.vi"("error in (no error)"=w1246) -> ("error out"=w1244:errorcluster)  [unwired: 1 out]
          }
          frame True {
          }
        }
      }
      frame "HW Close - Reserve 1", "HW Close - Reserve 2" {
        # "Place Holder"
      }
      frame "HW Close - SW" {
        n590 = stacked-sequence {
          frame #0 {
            # "Show Pages"
            n591 = property on="Main Tab" class="TabCtl (strict)"("Value"=enum32{"I/O Config", "Image"}."I/O Config" ("Main Tab")) -> ()  [unwired: 2 in, 2 out]
          }
          frame #1 {
            # "Update DAQ system state/status"
            n592 = call "Image-DO with Stage - System State.vi"("Set State (F:Get)"=TRUE ("Action (F:Get)"), "Sys State In"=Image-DO_with_Stage_-_Sys_State."HW Un_init") -> ()  [unwired: 7 in, 3 out]
          }
          frame #2 {
            w1260 = FALSE ("Scan")
            w1261 = FALSE ("Scan")
            # "Update GUI"
            n593 = property on="Connect" class="Bool (strict)"("Blinking"=w1261, "Value"=w1261) -> ()  [unwired: 2 in, 2 out]
            n594 = property on="Scan" class="Bool (strict)"("Blinking"=w1260, "Value"=w1260) -> ()  [unwired: 2 in, 2 out]
          }
        }
      }
      frame "Shutdown" {
        n595 = call "Image-DO with Stage - System State.vi"() -> ("Sys State Out"=w1262:T12)  [unwired: 9 in, 2 out]
        n596 = case shown="\"HW Un_init\"" w1262 {
          tunnel: [T9[] [{"Exec States"=enum."Exit", "U32"=0, "I32"=0, "DBL_1 (X)"=0.0, "DBL_2 (Y)"=0.0, "DBL_3 (Z)"=0.0, "Bool_1"=FALSE, "Bool_2"=FALSE, "Variant"=variant(string "")}] ("Actions") T9[] [{"Exec States"=enum."HW Close Crtl", "U32"=0, "I32"=0, "DBL_1 (X)"=0.0, "DBL_2 (Y)"=0.0, "DBL_3 (Z)"=0.0, "Bool_1"=FALSE, "Bool_2"=FALSE, "Variant"=variant(string "")}, {"Exec States"=enum."Exit", "U32"=0, "I32"=0, "DBL_1 (X)"=0.0, "DBL_2 (Y)"=0.0, "DBL_3 (Z)"=0.0, "Bool_1"=FALSE, "Bool_2"=FALSE, "Variant"=variant(string "")}] ("Actions") _] -> w1264
          frame "HW Un_init" {
            # "0: Exit"
          }
          frame "HW Initializing".."Configured" {
            # "0: HW Clost Ctrl\n1: Exit"
          }
          frame "Imaging".."Scanning" {
            # "Bad Call\nDon't exit while collecting data"
          }
        }
        n597 = call "Image-DO with Stage - Que Actions.vi"("Actions"=w1264, "Qqu Ref In"=w1266) -> ("Que Ref Out"=w1265:refnum<queue>)  [unwired: 8 in, 1 out]
      }
      frame "Error" {
        # "State\ncausing\nerror"
        # "Remove Error\nfrom Que"
        n598 = Dequeue Element(queue=w1280) -> (queue out=w1279:refnum<queue>)  [unwired: 2 in, 3 out]
        n599 = Unbundle By Name(w1275) -> ("source"=w1273:string, "code"=w1274:i32)
        n600 = Preview Queue Element(queue=w1279) -> (queue out=w1278:refnum<queue>, element=w1272:T9)  [unwired: 2 in, 2 out]
        n601 = case shown="Default" w1274 {
          tunnel: w1275 -> [w1292 _]
          tunnel: w1278 -> [w1286 w1294]
          tunnel: [w1286 w1294] -> w1277
          tunnel: w1273 -> [_ _]
          tunnel: w1272 -> [w1290 _]
          frame Default {
            w1291 = T31 0 items=["no dialog", "OK message", "continue or stop message", "OK message + warnings", "continue/stop + warnings"] ("type of dialog (OK msg:1)")
            n602 = Unbundle By Name(w1290) -> ("Exec States"=w1289:T10)
            n603 = call <vilib>:"General Error Handler.vi"("type of dialog (OK msg:1)"=w1291, "error in (no error)"=w1292) -> ("message"=w1288:string)  [unwired: 9 in, 4 out]
            n604 = Format Into String(format string="The program has skipped the current action due to the error listed below.  You can \"Ignore\" the error and proceed after a 10 second pause allowing time for front panel changes or \"Abort\" the application which is not recommended.  It may take a few rounds to clear all errors when exiting the program.\\n\\n\\nAction: \"%s\"\\n\\n%s", w1289, w1288) -> (resulting string=w1287:string)  [unwired: 2 in, 1 out]
            n605 = Two Button Dialog(message=w1287, 1:"Abort" ("T button name (\"OK\")"), 2:"Cancel" ("message")) -> (T button?=w1282:bool)
            n606 = case shown="False" w1282 {
              frame False {
                n607 = Stop() -> ()  [unwired: 1 in]
              }
              frame True {
                n608 = Wait (ms)(milliseconds to wait=u32 10000) -> ()  [unwired: 1 out]
              }
            }
          }
          frame 43 {
            # "User canceled action"
          }
        }
      }
      frame "Exit" {
        n609 = Quit LabVIEW(quit? (T)=w1295) -> ()
        n610 = property on="Main Tab" class="TabCtl (strict)"("Tabs Visible?"=TRUE) -> ()  [unwired: 2 in, 2 out]
        n611 = property on="Advance" class="Bool (strict)"("Visible"=TRUE, "DisabledEnum"=2) -> ()  [unwired: 2 in, 2 out]
      }
    }
    n612 = case shown="No Error" w289 {
      tunnel: w288 -> [w306 w309]
      tunnel: [w304 w308] -> w281
      frame No Error {
        n613 = Dequeue Element(queue=w306, timeout in ms (-1)=1) -> (queue out=w304:refnum<queue>)  [unwired: 1 in, 3 out]
      }
      frame Error {
        n614 = Enqueue Element At Opposite End(queue=w309, element=T9 {"Exec States"=enum."Error", "U32"=0, "I32"=0, "DBL_1 (X)"=0.0, "DBL_2 (Y)"=0.0, "DBL_3 (Z)"=0.0, "Bool_1"=FALSE, "Bool_2"=FALSE, "Variant"=variant(string "")}) -> (queue out=w308:refnum<queue>)  [unwired: 2 in, 2 out]
      }
    }
  }
  n615 = Release Queue(queue=w8, force destroy? (F)=TRUE, error in (no error)=w6) -> ()  [unwired: 3 out]
